vi "run_pharmaBotExpReliability_v0.002.vi"(0 "data in":T9={"daq_ao 1"="Dev1/ao0", "daq_ai 1"="Dev1/ai0", "experiment day folder"=path "C:/multiBot/patcherBot/data/temp", "Multiclamp init error"=0, "Multiclamp Handle Out"=6621140, "sampling rate (Hz)"=20000, "trial name"="t1"}, 5 "auto run?":bool, 7 "which manipulator":T10(ring), 9 "HEK/slice options":enum16{"slice", "HEK"}(ring), 11 "error in":errorcluster, 12 "common cluster":T6, 13 "individual controls in":T5, 14 "images":T3) -> (15 "error out":errorcluster)   [LabVIEW 2015]
uses:
  controls/Load and Save Controls_LV2009.llb/RWC_Actions.ctl
  wc_protocol_v1.003 Folder/whole_cell_protocol/Controls/clamp_profile.ctl
  controls/memtest_def.ctl
  Controls/Data.ctl
  wc_protocol_v1.003 Folder/whole_cell_protocol/Controls/cell_stats-v02.ctl
  pipette cleaning/pressure box/cleaning_soft/controls/actuator_type.ctl
  pipette cleaning/pressure box/cleaning_soft/controls/actuator_cluster.ctl
  machine_vision/coordinate model vis/transform_properties_actuators.ctl
  machine_vision/controls/transform_cluster_actuator.ctl
  controls/NH_method.ctl
  pipette cleaning/pressure box/cleaning_soft/controls/pressure_box_type.ctl
  pipette cleaning/pressure box/cleaning_soft/controls/pressure_box_control.ctl
  multipatch/controls/multipatch_common_controls_v4.ctl
  multipatch/controls/multipatch_individual_controls_v5.ctl
  <vilib>/vision/Image Controls.llb/IMAQ Image.ctl
  multipatch/controls/images_controls.ctl
panel:
  in  "PhaseX Cluster":T1
  out "Running":bool=TRUE
  out "Experiment Done":bool
  in  "Current Position":string
  out "Current Manipulator Position [uM]":i32[](array[numeric]) caption="Current Manipulator Position [um]" format="%.1f"
  in  "ExperimentOptionsCluster":T2
  out "HEK/slice options string":string
  out "config file":path=path "C:/multiBot/patcherBot/autoWCconfigs/autoWC_config_neuron-v07.ini"
  in  "load":bool
  in  "texts":enum32{"status", "comments", "release notes"}(tab)
  out "status":string
  in  "trial comments":string
  in  "release notes":string
  out "cell stats":T7 {"STD" format="%010.2f"; "Variance" format="%010.2f"; "Rt (MOhms)" format="%010.2f"; "tau (ms)" format="%08.2g"; "Cm (pF)" format="%08.2f"; "Ra (MOhms)" format="%010.2f"; "Rm (MOhms)" format="%010.2f"; "Ihold (pA)" format="%010.2f"}
  in  "save":bool
  in  "stop":bool
  in  "output":enum32{"VClamp", "IClamp"}(tab)
  out "Recorded currents (pA)":waveform(dbl)[](graph)
  out "Command steps (mV)":waveform(dbl)[](graph)
  out "Command steps (pA)":waveform(dbl)[](graph)
  out "Recorded voltage (mV)":waveform(dbl)[](graph)
  in  "run":bool
  in  "save as...":bool
  in  "update plots":bool
  in  "protocol creation":T8(tab)
  in  "DEBUG?":bool
  in  "auto WC run trigger":bool
  in  "twitter?":bool
  in  "protocol config":path=path "C:/multiBot/patcherBot/autoWCconfigs/autoWC_config_neuron-v07.ini"
  out "fast comp (pF)":dbl
  out "slow comp (pF)":dbl
  in  "Solution B":string="Wash"
  in  "V2 C Solution8":string="1:1 wash:H20"
  in  "V2 C Solution7":string
  in  "V2 C Solution6":string
  in  "V2 C Solution5":string
  in  "V2 C Solution4":string
  in  "V2 C Solution3":string
  in  "V2 C Solution2":string
  in  "V2 C Solution1":string
  in  "V1 A Solution8":string="1:1 wash:H20"
  in  "V1 A Solution7":string
  in  "V1 A Solution6":string
  in  "V1 A Solution5":string
  in  "V1 A Solution4":string
  in  "V1 A Solution3":string
  in  "V1 A Solution2":string="100uM Glu & 30uM Gly"
  in  "V1 A Solution1":string="Wash"
  in  "repMemTest set":enum32{"Iprot", "Vprot", "Imemtest", "Vmemtest"}(tab)
  out "repMemTest iprot cmd":waveform(dbl)[](graph)
  in  "repMemTest Iprot":T12={"Iclamp in"={"aLevel"=0.0, "aDelta"=0.0, "aDuration"=4000, "bLevel"=-200.0, "bDelta"=100.0, "bDuration"=4000, "cLevel"=0.0, "cDelta"=0.0, "cDuration"=4000}, "# iter"=6, "# reps IC"=1}
  out "repMemTest vprot cmd":waveform(dbl)[](graph)
  in  "repMemTest Vprot":T13={"Vclamp in"={"aLevel"=0.0, "aDelta"=0.0, "aDuration"=40000, "bLevel"=-30.0, "bDelta"=10.0, "bDuration"=40000, "cLevel"=0.0, "cDelta"=0.0, "cDuration"=40000}, "# iter"=8, "# reps VC"=1}
  out "repMemTest imemtest view":waveform(dbl)(graph)
  in  "repMemTest Iclamp memtest":T14={"Samples to Read"=2000, "Rate (Hz)"=20000.0, "Amplitude (mV/pA)"=-50.0, "Offset (mV/pA)"=0.0, "Frequency (Hz)"=10.0, "duty cycle (%)"=50.0, "phase"=0.0} {"phase" format="%.2p"; "duty cycle (%)" format="%0.2f"}
  out "repMemTest vmemtest view":waveform(dbl)(graph)
  in  "repMemTest Vclamp memtest":T14={"Samples to Read"=2000, "Rate (Hz)"=20000.0, "Amplitude (mV/pA)"=10.0, "Offset (mV/pA)"=0.0, "Frequency (Hz)"=10.0, "duty cycle (%)"=50.0, "phase"=-90.0} {"phase" format="%.2p"; "duty cycle (%)" format="%0.2f"}
  in  "wait after init (s)":dbl=0.1
  in  "repMemTest sets":T15={" Iprot"=FALSE, " Vprot"=FALSE, " Imemtest"=FALSE, " Vmemtest"=TRUE}
  in  "wait after repMemTest set (s)":dbl=0.1
  in  "Experimental Phases":T16(tab)
  in  "PhaseA Experiment Option":string(combo)="Single Jump"
  in  "Experiment Selection A":T17(tab)
  in  "Single Jump A":T18={"Which Position to use for Experiment"=enum."Jumper Position B-A", "Start Position (N)"="Jumper Posistion B", "Jump Position (m)"="Jumper Posistion A", "Duration (s)"=10.0, "Delay (s)"=1.0, "Pulse Width (s)"=1.0, "Valve 1 Position"=2, "Valve 2 Position"=2, "Replicates"=1.0, "Vholding (mV)"=-60.0} {"Replicates" min=1.0; "Valve 2 Position" min=1 max=8; "Valve 1 Position" min=1 max=8}
  in  "Solution Change A":T19={"Which Position to use for Experiment"=enum."Jumper Safe Position", "Duration (s)"=0.0, "Delay (s)"=0.0, "Pulse Width (s)"=0.0, "Valve Start Position"=1, "Valve Jump Position"=1, "Replicates"=1.0, "Vholding (mV)"=0.0} {"Replicates" min=1.0; "Valve Jump Position" min=1 max=8; "Valve Start Position" min=1 max=8}
  in  "Voltage Step A":T20={"Which Position to use for Experiment"=enum."Jumper Safe Position", "Duration (s)"=0.0, "Delay (s)"=0.0, "Step Width (s)"=0.0, "Voltage Start (mV)"=1, "Voltage Step (mV)"=1, "Replicates"=1.0, "Voltage End (mV)"=1, "Number of Step"=0.0, "Valve Position"=1, "Vholding (mV)"=0.0} {"Valve Position" min=1 max=8; "Voltage End (mV)" min=1 max=8; "Replicates" min=1.0; "Voltage Step (mV)" min=1 max=8; "Voltage Start (mV)" min=1 max=8}
  in  "Voltage Ramp A":T21={"Which Position to use for Experiment"=enum."Jumper Safe Position", "Duration (s)"=0.0, "Delay (s)"=0.0, "Ramp Slope (mV/s)"=0.0, "Voltage Start (mV)"=1, "Replicates"=1.0, "Voltage End (mV)"=1, "Ramp Duration (s)"=0.0, "Valve Position"=1, "Vholding (mV)"=0.0} {"Valve Position" min=1 max=8; "Voltage End (mV)" min=1 max=8; "Replicates" min=1.0; "Voltage Start (mV)" min=1 max=8}
  in  "Jump Train A":T22={"Which Position to use for Experiment"=enum."Jumper Safe Position", "Start Position (N)"="", "Jump Position (m)"="", "Duration (s)"=0.0, "Delay (s)"=0.0, "Pulse Width (s)"=0.0, "Valve 1 Position"=1, "Valve 2 Position"=1, "Replicates"=1.0, "Pulse Period (s)"=0.0, "Vholding (mV)"=1.0} {"Vholding (mV)" min=1.0; "Replicates" min=1.0; "Valve 2 Position" min=1 max=8; "Valve 1 Position" min=1 max=8}
  in  "Paired Pulse A":T23={"Which Position to use for Experiment"=enum."Jumper Safe Position", "Start Position (N)"="", "Jump Position (m)"="", "Duration (s)"=0.0, "Delay (s)"=0.0, "Pulse Width (s)"=0.0, "Valve 1 Position"=1, "Valve 2 Position"=1, "Replicates"=1.0, "Pulse Delay (s)"=0.0, "Pulse Delta Delay (s)"=0.0, "Vholding (mV)"=0.0} {"Replicates" min=1.0; "Valve 2 Position" min=1 max=8; "Valve 1 Position" min=1 max=8}
  in  "Single Manip Jump A":T24={"Start Position (N)"=enum."Jumper Safe Position", "Duration (s)"=0.0, "Delay (s)"=0.0, "Pulse Width (s)"=0.0, "Valve 1 Position"=1, "Valve 2 Position"=1, "Replicates"=1.0, "Jump Position (m)"=enum."Jumper Safe Position", "Vholding (mV)"=0.0} {"Replicates" min=1.0; "Valve 2 Position" min=1 max=8; "Valve 1 Position" min=1 max=8}
  in  "PhaseB Experiment Option":string(combo)="Single Jump"
  in  "Experiment Selection B":T17(tab)
  in  "Single Jump B":T18={"Which Position to use for Experiment"=enum."Jumper Position B-A", "Start Position (N)"="Jumper Posistion B", "Jump Position (m)"="Jumper Posistion A", "Duration (s)"=10.0, "Delay (s)"=1.0, "Pulse Width (s)"=1.0, "Valve 1 Position"=2, "Valve 2 Position"=2, "Replicates"=1.0, "Vholding (mV)"=40.0} {"Replicates" min=1.0; "Valve 2 Position" min=1 max=8; "Valve 1 Position" min=1 max=8}
  in  "Solution Change B":T19={"Which Position to use for Experiment"=enum."Jumper Safe Position", "Duration (s)"=0.0, "Delay (s)"=0.0, "Pulse Width (s)"=0.0, "Valve Start Position"=1, "Valve Jump Position"=1, "Replicates"=1.0, "Vholding (mV)"=0.0} {"Replicates" min=1.0; "Valve Jump Position" min=1 max=8; "Valve Start Position" min=1 max=8}
  in  "Voltage Step B":T20={"Which Position to use for Experiment"=enum."Jumper Safe Position", "Duration (s)"=0.0, "Delay (s)"=0.0, "Step Width (s)"=0.0, "Voltage Start (mV)"=1, "Voltage Step (mV)"=1, "Replicates"=1.0, "Voltage End (mV)"=1, "Number of Step"=0.0, "Valve Position"=1, "Vholding (mV)"=0.0} {"Valve Position" min=1 max=8; "Voltage End (mV)" min=1 max=8; "Replicates" min=1.0; "Voltage Step (mV)" min=1 max=8; "Voltage Start (mV)" min=1 max=8}
  in  "Voltage Ramp B":T21={"Which Position to use for Experiment"=enum."Jumper Safe Position", "Duration (s)"=0.0, "Delay (s)"=0.0, "Ramp Slope (mV/s)"=0.0, "Voltage Start (mV)"=1, "Replicates"=1.0, "Voltage End (mV)"=1, "Ramp Duration (s)"=0.0, "Valve Position"=1, "Vholding (mV)"=0.0} {"Valve Position" min=1 max=8; "Voltage End (mV)" min=1 max=8; "Replicates" min=1.0; "Voltage Start (mV)" min=1 max=8}
  in  "Jump Train B":T22={"Which Position to use for Experiment"=enum."Jumper Safe Position", "Start Position (N)"="", "Jump Position (m)"="", "Duration (s)"=0.0, "Delay (s)"=0.0, "Pulse Width (s)"=0.0, "Valve 1 Position"=1, "Valve 2 Position"=1, "Replicates"=1.0, "Pulse Period (s)"=0.0, "Vholding (mV)"=1.0} {"Vholding (mV)" min=1.0; "Replicates" min=1.0; "Valve 2 Position" min=1 max=8; "Valve 1 Position" min=1 max=8}
  in  "Paired Pulse B":T23={"Which Position to use for Experiment"=enum."Jumper Safe Position", "Start Position (N)"="", "Jump Position (m)"="", "Duration (s)"=0.0, "Delay (s)"=0.0, "Pulse Width (s)"=0.0, "Valve 1 Position"=1, "Valve 2 Position"=1, "Replicates"=1.0, "Pulse Delay (s)"=0.0, "Pulse Delta Delay (s)"=0.0, "Vholding (mV)"=0.0} {"Replicates" min=1.0; "Valve 2 Position" min=1 max=8; "Valve 1 Position" min=1 max=8}
  in  "Single Manip Jump B":T24={"Start Position (N)"=enum."Jumper Safe Position", "Duration (s)"=0.0, "Delay (s)"=0.0, "Pulse Width (s)"=0.0, "Valve 1 Position"=1, "Valve 2 Position"=1, "Replicates"=1.0, "Jump Position (m)"=enum."Jumper Safe Position", "Vholding (mV)"=0.0} {"Replicates" min=1.0; "Valve 2 Position" min=1 max=8; "Valve 1 Position" min=1 max=8}
  in  "PhaseC Experiment Option":string(combo)="Single Manip Jump"
  in  "Experiment Selection C":T17(tab)=enum."Single Manip Jump"
  in  "Single Jump C":T18={"Which Position to use for Experiment"=enum."Jumper Safe Position", "Start Position (N)"="", "Jump Position (m)"="", "Duration (s)"=0.0, "Delay (s)"=0.0, "Pulse Width (s)"=0.0, "Valve 1 Position"=1, "Valve 2 Position"=1, "Replicates"=1.0, "Vholding (mV)"=0.0} {"Replicates" min=1.0; "Valve 2 Position" min=1 max=8; "Valve 1 Position" min=1 max=8}
  in  "Solution Change C":T19={"Which Position to use for Experiment"=enum."Jumper Safe Position", "Duration (s)"=0.0, "Delay (s)"=0.0, "Pulse Width (s)"=0.0, "Valve Start Position"=1, "Valve Jump Position"=1, "Replicates"=1.0, "Vholding (mV)"=0.0} {"Replicates" min=1.0; "Valve Jump Position" min=1 max=8; "Valve Start Position" min=1 max=8}
  in  "Voltage Step C":T20={"Which Position to use for Experiment"=enum."Jumper Safe Position", "Duration (s)"=0.0, "Delay (s)"=0.0, "Step Width (s)"=0.0, "Voltage Start (mV)"=1, "Voltage Step (mV)"=1, "Replicates"=1.0, "Voltage End (mV)"=1, "Number of Step"=0.0, "Valve Position"=1, "Vholding (mV)"=0.0} {"Valve Position" min=1 max=8; "Voltage End (mV)" min=1 max=8; "Replicates" min=1.0; "Voltage Step (mV)" min=1 max=8; "Voltage Start (mV)" min=1 max=8}
  in  "Voltage Ramp C":T21={"Which Position to use for Experiment"=enum."Jumper Safe Position", "Duration (s)"=0.0, "Delay (s)"=0.0, "Ramp Slope (mV/s)"=0.0, "Voltage Start (mV)"=1, "Replicates"=1.0, "Voltage End (mV)"=1, "Ramp Duration (s)"=0.0, "Valve Position"=1, "Vholding (mV)"=0.0} {"Valve Position" min=1 max=8; "Voltage End (mV)" min=1 max=8; "Replicates" min=1.0; "Voltage Start (mV)" min=1 max=8}
  in  "Jump Train C":T22={"Which Position to use for Experiment"=enum."Jumper Safe Position", "Start Position (N)"="", "Jump Position (m)"="", "Duration (s)"=0.0, "Delay (s)"=0.0, "Pulse Width (s)"=0.0, "Valve 1 Position"=1, "Valve 2 Position"=1, "Replicates"=1.0, "Pulse Period (s)"=0.0, "Vholding (mV)"=1.0} {"Vholding (mV)" min=1.0; "Replicates" min=1.0; "Valve 2 Position" min=1 max=8; "Valve 1 Position" min=1 max=8}
  in  "Paired Pulse C":T23={"Which Position to use for Experiment"=enum."Jumper Safe Position", "Start Position (N)"="", "Jump Position (m)"="", "Duration (s)"=0.0, "Delay (s)"=0.0, "Pulse Width (s)"=0.0, "Valve 1 Position"=1, "Valve 2 Position"=1, "Replicates"=1.0, "Pulse Delay (s)"=0.0, "Pulse Delta Delay (s)"=0.0, "Vholding (mV)"=0.0} {"Replicates" min=1.0; "Valve 2 Position" min=1 max=8; "Valve 1 Position" min=1 max=8}
  in  "Single Manip Jump C":T24={"Start Position (N)"=enum."Jumper Position B", "Duration (s)"=10.0, "Delay (s)"=1.0, "Pulse Width (s)"=1.0, "Valve 1 Position"=2, "Valve 2 Position"=2, "Replicates"=1.0, "Jump Position (m)"=enum."Jumper Position A", "Vholding (mV)"=40.0} {"Replicates" min=1.0; "Valve 2 Position" min=1 max=8; "Valve 1 Position" min=1 max=8}
  in  "PhaseD Experiment Option":string(combo)="Single Manip Jump"
  in  "Experiment Selection D":T17(tab)=enum."Single Manip Jump"
  in  "Single Jump D":T18={"Which Position to use for Experiment"=enum."Jumper Safe Position", "Start Position (N)"="", "Jump Position (m)"="", "Duration (s)"=0.0, "Delay (s)"=0.0, "Pulse Width (s)"=0.0, "Valve 1 Position"=1, "Valve 2 Position"=1, "Replicates"=1.0, "Vholding (mV)"=0.0} {"Replicates" min=1.0; "Valve 2 Position" min=1 max=8; "Valve 1 Position" min=1 max=8}
  in  "Solution Change D":T19={"Which Position to use for Experiment"=enum."Jumper Safe Position", "Duration (s)"=0.0, "Delay (s)"=0.0, "Pulse Width (s)"=0.0, "Valve Start Position"=1, "Valve Jump Position"=1, "Replicates"=1.0, "Vholding (mV)"=0.0} {"Replicates" min=1.0; "Valve Jump Position" min=1 max=8; "Valve Start Position" min=1 max=8}
  in  "Voltage Step D":T20={"Which Position to use for Experiment"=enum."Jumper Safe Position", "Duration (s)"=0.0, "Delay (s)"=0.0, "Step Width (s)"=0.0, "Voltage Start (mV)"=1, "Voltage Step (mV)"=1, "Replicates"=1.0, "Voltage End (mV)"=1, "Number of Step"=0.0, "Valve Position"=1, "Vholding (mV)"=0.0} {"Valve Position" min=1 max=8; "Voltage End (mV)" min=1 max=8; "Replicates" min=1.0; "Voltage Step (mV)" min=1 max=8; "Voltage Start (mV)" min=1 max=8}
  in  "Voltage Ramp D":T21={"Which Position to use for Experiment"=enum."Jumper Safe Position", "Duration (s)"=0.0, "Delay (s)"=0.0, "Ramp Slope (mV/s)"=0.0, "Voltage Start (mV)"=1, "Replicates"=1.0, "Voltage End (mV)"=1, "Ramp Duration (s)"=0.0, "Valve Position"=1, "Vholding (mV)"=0.0} {"Valve Position" min=1 max=8; "Voltage End (mV)" min=1 max=8; "Replicates" min=1.0; "Voltage Start (mV)" min=1 max=8}
  in  "Jump Train D":T22={"Which Position to use for Experiment"=enum."Jumper Safe Position", "Start Position (N)"="", "Jump Position (m)"="", "Duration (s)"=0.0, "Delay (s)"=0.0, "Pulse Width (s)"=0.0, "Valve 1 Position"=1, "Valve 2 Position"=1, "Replicates"=1.0, "Pulse Period (s)"=0.0, "Vholding (mV)"=1.0} {"Vholding (mV)" min=1.0; "Replicates" min=1.0; "Valve 2 Position" min=1 max=8; "Valve 1 Position" min=1 max=8}
  in  "Paired Pulse D":T23={"Which Position to use for Experiment"=enum."Jumper Safe Position", "Start Position (N)"="", "Jump Position (m)"="", "Duration (s)"=0.0, "Delay (s)"=0.0, "Pulse Width (s)"=0.0, "Valve 1 Position"=1, "Valve 2 Position"=1, "Replicates"=1.0, "Pulse Delay (s)"=0.0, "Pulse Delta Delay (s)"=0.0, "Vholding (mV)"=0.0} {"Replicates" min=1.0; "Valve 2 Position" min=1 max=8; "Valve 1 Position" min=1 max=8}
  in  "Single Manip Jump D":T24={"Start Position (N)"=enum."Jumper Position B", "Duration (s)"=10.0, "Delay (s)"=1.0, "Pulse Width (s)"=1.0, "Valve 1 Position"=2, "Valve 2 Position"=2, "Replicates"=1.0, "Jump Position (m)"=enum."Jumper Position A", "Vholding (mV)"=-60.0} {"Replicates" min=1.0; "Valve 2 Position" min=1 max=8; "Valve 1 Position" min=1 max=8}
  in  "PhaseE Experiment Option":string(combo)="Single Manip Jump"
  in  "Experiment Selection E":T17(tab)=enum."Single Manip Jump"
  in  "Single Jump E":T18={"Which Position to use for Experiment"=enum."Jumper Safe Position", "Start Position (N)"="", "Jump Position (m)"="", "Duration (s)"=0.0, "Delay (s)"=0.0, "Pulse Width (s)"=0.0, "Valve 1 Position"=1, "Valve 2 Position"=1, "Replicates"=1.0, "Vholding (mV)"=0.0} {"Replicates" min=1.0; "Valve 2 Position" min=1 max=8; "Valve 1 Position" min=1 max=8}
  in  "Solution Change E":T19={"Which Position to use for Experiment"=enum."Jumper Safe Position", "Duration (s)"=0.0, "Delay (s)"=0.0, "Pulse Width (s)"=0.0, "Valve Start Position"=1, "Valve Jump Position"=1, "Replicates"=1.0, "Vholding (mV)"=0.0} {"Replicates" min=1.0; "Valve Jump Position" min=1 max=8; "Valve Start Position" min=1 max=8}
  in  "Voltage Step E":T20={"Which Position to use for Experiment"=enum."Jumper Safe Position", "Duration (s)"=0.0, "Delay (s)"=0.0, "Step Width (s)"=0.0, "Voltage Start (mV)"=1, "Voltage Step (mV)"=1, "Replicates"=1.0, "Voltage End (mV)"=1, "Number of Step"=0.0, "Valve Position"=1, "Vholding (mV)"=0.0} {"Valve Position" min=1 max=8; "Voltage End (mV)" min=1 max=8; "Replicates" min=1.0; "Voltage Step (mV)" min=1 max=8; "Voltage Start (mV)" min=1 max=8}
  in  "Voltage Ramp E":T21={"Which Position to use for Experiment"=enum."Jumper Safe Position", "Duration (s)"=0.0, "Delay (s)"=0.0, "Ramp Slope (mV/s)"=0.0, "Voltage Start (mV)"=1, "Replicates"=1.0, "Voltage End (mV)"=1, "Ramp Duration (s)"=0.0, "Valve Position"=1, "Vholding (mV)"=0.0} {"Valve Position" min=1 max=8; "Voltage End (mV)" min=1 max=8; "Replicates" min=1.0; "Voltage Start (mV)" min=1 max=8}
  in  "Jump Train E":T22={"Which Position to use for Experiment"=enum."Jumper Safe Position", "Start Position (N)"="", "Jump Position (m)"="", "Duration (s)"=0.0, "Delay (s)"=0.0, "Pulse Width (s)"=0.0, "Valve 1 Position"=1, "Valve 2 Position"=1, "Replicates"=1.0, "Pulse Period (s)"=0.0, "Vholding (mV)"=1.0} {"Vholding (mV)" min=1.0; "Replicates" min=1.0; "Valve 2 Position" min=1 max=8; "Valve 1 Position" min=1 max=8}
  in  "Paired Pulse E":T23={"Which Position to use for Experiment"=enum."Jumper Safe Position", "Start Position (N)"="", "Jump Position (m)"="", "Duration (s)"=0.0, "Delay (s)"=0.0, "Pulse Width (s)"=0.0, "Valve 1 Position"=1, "Valve 2 Position"=1, "Replicates"=1.0, "Pulse Delay (s)"=0.0, "Pulse Delta Delay (s)"=0.0, "Vholding (mV)"=0.0} {"Replicates" min=1.0; "Valve 2 Position" min=1 max=8; "Valve 1 Position" min=1 max=8}
  in  "Single Manip Jump E":T24={"Start Position (N)"=enum."Jumper Position B", "Duration (s)"=10.0, "Delay (s)"=1.0, "Pulse Width (s)"=1.0, "Valve 1 Position"=2, "Valve 2 Position"=2, "Replicates"=1.0, "Jump Position (m)"=enum."Jumper Position o-A", "Vholding (mV)"=-60.0} {"Replicates" min=1.0; "Valve 2 Position" min=1 max=8; "Valve 1 Position" min=1 max=8}
  in  "PhaseF Experiment Option":string(combo)="Single Jump"
  in  "Experiment Selection F":T17(tab)
  in  "Single Jump F":T18={"Which Position to use for Experiment"=enum."Jumper Position B-A", "Start Position (N)"="Jumper Posistion B", "Jump Position (m)"="Jumper Posistion A", "Duration (s)"=10.0, "Delay (s)"=1.0, "Pulse Width (s)"=1.0, "Valve 1 Position"=2, "Valve 2 Position"=2, "Replicates"=1.0, "Vholding (mV)"=-60.0} {"Replicates" min=1.0; "Valve 2 Position" min=1 max=8; "Valve 1 Position" min=1 max=8}
  in  "Solution Change F":T19={"Which Position to use for Experiment"=enum."Jumper Safe Position", "Duration (s)"=0.0, "Delay (s)"=0.0, "Pulse Width (s)"=0.0, "Valve Start Position"=1, "Valve Jump Position"=1, "Replicates"=1.0, "Vholding (mV)"=0.0} {"Replicates" min=1.0; "Valve Jump Position" min=1 max=8; "Valve Start Position" min=1 max=8}
  in  "Voltage Step F":T20={"Which Position to use for Experiment"=enum."Jumper Safe Position", "Duration (s)"=0.0, "Delay (s)"=0.0, "Step Width (s)"=0.0, "Voltage Start (mV)"=1, "Voltage Step (mV)"=1, "Replicates"=1.0, "Voltage End (mV)"=1, "Number of Step"=0.0, "Valve Position"=1, "Vholding (mV)"=0.0} {"Valve Position" min=1 max=8; "Voltage End (mV)" min=1 max=8; "Replicates" min=1.0; "Voltage Step (mV)" min=1 max=8; "Voltage Start (mV)" min=1 max=8}
  in  "Voltage Ramp F":T21={"Which Position to use for Experiment"=enum."Jumper Safe Position", "Duration (s)"=0.0, "Delay (s)"=0.0, "Ramp Slope (mV/s)"=0.0, "Voltage Start (mV)"=1, "Replicates"=1.0, "Voltage End (mV)"=1, "Ramp Duration (s)"=0.0, "Valve Position"=1, "Vholding (mV)"=0.0} {"Valve Position" min=1 max=8; "Voltage End (mV)" min=1 max=8; "Replicates" min=1.0; "Voltage Start (mV)" min=1 max=8}
  in  "Jump Train F":T22={"Which Position to use for Experiment"=enum."Jumper Safe Position", "Start Position (N)"="", "Jump Position (m)"="", "Duration (s)"=0.0, "Delay (s)"=0.0, "Pulse Width (s)"=0.0, "Valve 1 Position"=1, "Valve 2 Position"=1, "Replicates"=1.0, "Pulse Period (s)"=0.0, "Vholding (mV)"=1.0} {"Vholding (mV)" min=1.0; "Replicates" min=1.0; "Valve 2 Position" min=1 max=8; "Valve 1 Position" min=1 max=8}
  in  "Paired Pulse F":T23={"Which Position to use for Experiment"=enum."Jumper Safe Position", "Start Position (N)"="", "Jump Position (m)"="", "Duration (s)"=0.0, "Delay (s)"=0.0, "Pulse Width (s)"=0.0, "Valve 1 Position"=1, "Valve 2 Position"=1, "Replicates"=1.0, "Pulse Delay (s)"=0.0, "Pulse Delta Delay (s)"=0.0, "Vholding (mV)"=0.0} {"Replicates" min=1.0; "Valve 2 Position" min=1 max=8; "Valve 1 Position" min=1 max=8}
  in  "Single Manip Jump F":T24={"Start Position (N)"=enum."Jumper Safe Position", "Duration (s)"=0.0, "Delay (s)"=0.0, "Pulse Width (s)"=0.0, "Valve 1 Position"=1, "Valve 2 Position"=1, "Replicates"=1.0, "Jump Position (m)"=enum."Jumper Safe Position", "Vholding (mV)"=0.0} {"Replicates" min=1.0; "Valve 2 Position" min=1 max=8; "Valve 1 Position" min=1 max=8}
  in  "ending set":enum32{"Iprot", "Vprot", "Imemtest", "Vmemtest"}(tab)
  in  "holding memtest":bool=TRUE
  in  "holding set":enum32{"VClamp", "IClamp"}(tab)
  out "holding vmemtest cmd":waveform(dbl)(graph)
  in  "holding Vclamp memtest":T14={"Samples to Read"=2000, "Rate (Hz)"=20000.0, "Amplitude (mV/pA)"=10.0, "Offset (mV/pA)"=0.0, "Frequency (Hz)"=10.0, "duty cycle (%)"=50.0, "phase"=-90.0} {"phase" format="%.2p"; "duty cycle (%)" format="%0.2f"}
  out "holding imemtest cmd":waveform(dbl)(graph)
  in  "holding Iclamp memtest":T14={"Samples to Read"=2000, "Rate (Hz)"=20000.0, "Amplitude (mV/pA)"=-50.0, "Offset (mV/pA)"=0.0, "Frequency (Hz)"=10.0, "duty cycle (%)"=50.0, "phase"=0.0} {"phase" format="%.2p"; "duty cycle (%)" format="%0.2f"}
  # "IClamp step protocol"
  # "x"
  # "VClamp step protocol"
  # "x"
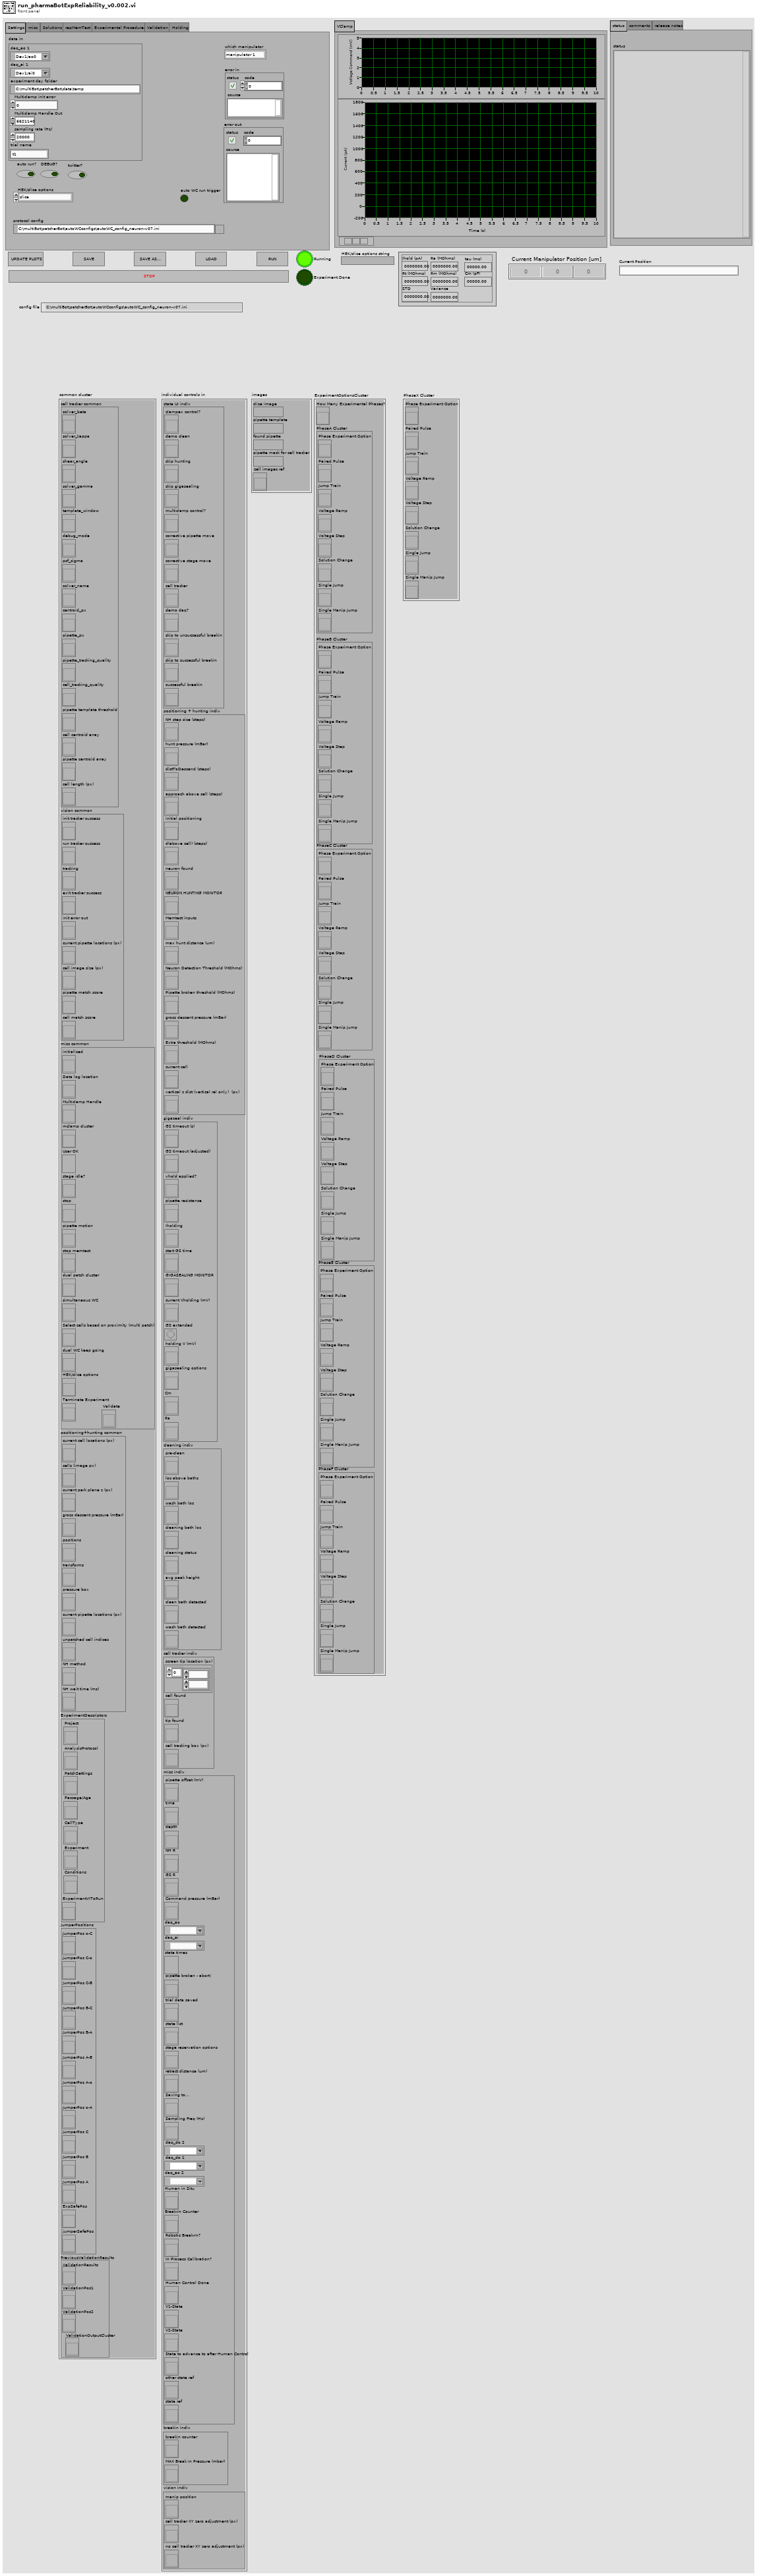
[diagram p1: front panel]
types:
  T1 = cluster{"Phase Experiment Option":refnum<vi>, "Paired Pulse":refnum<vi>, "Jump Train":refnum<vi>, "Voltage Ramp":refnum<vi>, "Voltage Step":refnum<vi>, "Solution Change":refnum<vi>, "Single Jump":refnum<vi>, "Single Manip Jump":refnum<vi>}
  T2 = cluster{"How Many Experimental Phases?":refnum<vi>, "PhaseA Cluster":cluster{"Phase Experiment Option":refnum<vi>, "Paired Pulse":refnum<vi>, "Jump Train":refnum<vi>, "Voltage Ramp":refnum<vi>, "Voltage Step":refnum<vi>, "Solution Change":refnum<vi>, "Single Jump":refnum<vi>, "Single Manip Jump":refnum<vi>}, "PhaseB Cluster":cluster{"Phase Experiment Option":refnum<vi>, "Paired Pulse":refnum<vi>, "Jump Train":refnum<vi>, "Voltage Ramp":refnum<vi>, "Voltage Step":refnum<vi>, "Solution Change":refnum<vi>, "Single Jump":refnum<vi>, "Single Manip Jump":refnum<vi>}, "PhaseC Cluster":cluster{"Phase Experiment Option":refnum<vi>, "Paired Pulse":refnum<vi>, "Jump Train":refnum<vi>, "Voltage Ramp":refnum<vi>, "Voltage Step":refnum<vi>, "Solution Change":refnum<vi>, "Single Jump":refnum<vi>, "Single Manip Jump":refnum<vi>}, "PhaseD Cluster":cluster{"Phase Experiment Option":refnum<vi>, "Paired Pulse":refnum<vi>, "Jump Train":refnum<vi>, "Voltage Ramp":refnum<vi>, "Voltage Step":refnum<vi>, "Solution Change":refnum<vi>, "Single Jump":refnum<vi>, "Single Manip Jump":refnum<vi>}, "PhaseE Cluster":cluster{"Phase Experiment Option":refnum<vi>, "Paired Pulse":refnum<vi>, "Jump Train":refnum<vi>, "Voltage Ramp":refnum<vi>, "Voltage Step":refnum<vi>, "Solution Change":refnum<vi>, "Single Jump":refnum<vi>, "Single Manip Jump":refnum<vi>}, "PhaseF Cluster":cluster{"Phase Experiment Option":refnum<vi>, "Paired Pulse":refnum<vi>, "Jump Train":refnum<vi>, "Voltage Ramp":refnum<vi>, "Voltage Step":refnum<vi>, "Solution Change":refnum<vi>, "Single Jump":refnum<vi>, "Single Manip Jump":refnum<vi>}}
  T3 = typedef "images_controls.ctl" = cluster{"slice image":T4, "pipette template":T4, "found pipette":T4, "pipette mask for cell tracker":T4, "cell images ref":refnum<vi>}
  T4 = typedef "IMAQ Image.ctl" = refnum<image>
  T5 = typedef "multipatch_individual_controls_v5.ctl" = cluster{"state UI indiv":cluster{"clampex control?":refnum<vi>, "demo clean":refnum<vi>, "skip hunting":refnum<vi>, "skip gigasealing":refnum<vi>, "multiclamp control?":refnum<vi>, "corrective pipette move":refnum<vi>, "corrective stage move":refnum<vi>, "cell tracker":refnum<vi>, "demo daq?":refnum<vi>, "skip to unsuccessful breakin":refnum<vi>, "skip to successful breakin":refnum<vi>, "successful breakin":refnum<vi>}, "positioning + hunting indiv":cluster{"NH step size (steps)":refnum<vi>, "hunt pressure (mBar)":refnum<vi>, "distToDescend (steps)":refnum<vi>, "approach above cell (steps)":refnum<vi>, "initial positioning":refnum<vi>, "d(above cell) (steps)":refnum<vi>, "neuron found":refnum<vi>, "NEURON HUNTING MONITOR":refnum<vi>, "Memtest inputs":refnum<vi>, "max hunt distance (um)":refnum<vi>, "Neuron Detection Threshold (MOhms)":refnum<vi>, "Pipette broken threshold (MOhms)":refnum<vi>, "gross descent pressure (mBar)":refnum<vi>, "Extra threshold (MOhms)":refnum<vi>, "current cell":refnum<vi>, "vertical z dist (vertical rel only)  (px)":refnum<vi>}, "gigaseal indiv":cluster{"GS timeout (s)":refnum<vi>, "GS timeout (adjusted)":refnum<vi>, "vhold applied?":refnum<vi>, "pipette resistance":refnum<vi>, "Iholding":refnum<vi>, "start GS time":refnum<vi>, "GIGASEALING MONITOR":refnum<vi>, "current Vholding (mV)":refnum<vi>, "GS extended":refnum<vi>, "holding V (mV)":refnum<vi>, "gigasealing options":refnum<vi>, "Cm":refnum<vi>, "Ra ":refnum<vi>}, "cleaning indiv":cluster{"pre-clean":refnum<vi>, "loc above baths":refnum<vi>, "wash bath loc":refnum<vi>, "cleaning bath loc":refnum<vi>, "cleaning status":refnum<vi>, "avg peak height":refnum<vi>, "clean bath detected":refnum<vi>, "wash bath detected":refnum<vi>}, "cell tracker indiv":cluster{"screen tip location (px)":refnum<vi>, "cell found":refnum<vi>, "tip found":refnum<vi>, "cell tracking box (px)":refnum<vi>}, "misc indiv":cluster{"pipette offset (mV)":refnum<vi>, "time":refnum<vi>, "depth":refnum<vi>, "NH R":refnum<vi>, "GS R":refnum<vi>, "Command pressure (mBar)":refnum<vi>, "daq_ao":tag, "daq_ai":tag, "state times":refnum<vi>, "pipette broken - abort!":refnum<vi>, "trial data saved":refnum<vi>, "state list":refnum<vi>, "stage reservation options":refnum<vi>, "retract distance (um)":refnum<vi>, "Saving to...":refnum<vi>, "Sampling Freq (Hz)":refnum<vi>, "daq_do 2":tag, "daq_do 1":tag, "daq_ao 2":tag, "Human in Situ":refnum<vi>, "Break-In Counter":refnum<vi>, "Robotic Break-In?":refnum<vi>, "In Process Calibration?":refnum<vi>, "Human Control Done":refnum<vi>, "V1-State":refnum<vi>, "V2-State":refnum<vi>, "State to advance to after Human Control":refnum<vi>, "other state ref":refnum<vi>, "state ref":refnum<vi>}, "breakin indiv":cluster{"breakin counter":refnum<vi>, "MAX Break In Pressure (mbar)":refnum<vi>}, "vision indiv":cluster{"manip position":refnum<vi>, "cell tracker XY zero adjustment (px)":refnum<vi>, "no cell tracker XY zero adjustment (px)":refnum<vi>}}
  T6 = typedef "multipatch_common_controls_v4.ctl" = cluster{"cell tracker common":cluster{"solver_beta":refnum<vi>, "solver_kappa":refnum<vi>, "shear_angle":refnum<vi>, "solver_gamma":refnum<vi>, "template_window":refnum<vi>, "debug_mode":refnum<vi>, "psf_sigma":refnum<vi>, "solver_name":refnum<vi>, "centroid_px":refnum<vi>, "pipette_px":refnum<vi>, "pipette_tracking_quality":refnum<vi>, "cell_tracking_quality":refnum<vi>, "pipette template threshold":refnum<vi>, "cell centroid array":refnum<vi>, "pipette centroid array":refnum<vi>, "cell length (px)":refnum<vi>}, "vision common":cluster{"init tracker success":refnum<vi>, "run tracker success":refnum<vi>, "tracking":refnum<vi>, "exit tracker success":refnum<vi>, "init error out":refnum<vi>, "current pipette locations (px)":refnum<vi>, "cell image size (px)":refnum<vi>, "pipette match score":refnum<vi>, "cell match score":refnum<vi>}, "misc common":cluster{"initialized":refnum<vi>, "Data log location":refnum<vi>, "Multiclamp Handle":refnum<vi>, "mclamp cluster":refnum<vi>, "User OK":refnum<vi>, "stage idle?":refnum<vi>, "stop":refnum<vi>, "pipette motion":refnum<vi>, "stop memtest":refnum<vi>, "dual patch cluster":refnum<vi>, "simultaneous WC":refnum<vi>, "Select cells based on proximity (multi patch)":refnum<vi>, "dual WC keep going":refnum<vi>, "HEK/slice options":refnum<vi>, "Terminate Experiment":refnum<vi>, "Validate":refnum<vi>}, "positioning+hunting common":cluster{"current cell locations (px)":refnum<vi>, "cells (image px)":refnum<vi>, "current park plane z (px)":refnum<vi>, "gross descent pressure (mBar)":refnum<vi>, "positions":refnum<vi>, "transforms":refnum<vi>, "pressure box":refnum<vi>, "current pipette locations (px)":refnum<vi>, "unpatched cell indices":refnum<vi>, "NH method":refnum<vi>, "NH wait time (ms)":refnum<vi>}, "ExperimentDescriptors":cluster{"Project":refnum<vi>, "AnalysisProtocol":refnum<vi>, "PatchSettings":refnum<vi>, "Passage/Age":refnum<vi>, "CellType":refnum<vi>, "Experiment":refnum<vi>, "Conditions":refnum<vi>, "ExperimentVIToRun":refnum<vi>}, "JumperPositions":cluster{"JumperPos o-C":refnum<vi>, "JumperPos C-o":refnum<vi>, "JumperPos C-B":refnum<vi>, "JumperPos B-C":refnum<vi>, "JumperPos B-A":refnum<vi>, "JumperPos A-B":refnum<vi>, "JumperPos A-o":refnum<vi>, "JumperPos o-A":refnum<vi>, "JumperPos C":refnum<vi>, "JumperPos B":refnum<vi>, "JumperPos A":refnum<vi>, "ExpSafePos":refnum<vi>, "jumperSafePos":refnum<vi>}, "PreviousValidationResults":cluster{"ValidationResults":refnum<vi>, "ValidationPos1":refnum<vi>, "ValidationPos2":refnum<vi>, "ValidationOutputCluster":refnum<vi>}}
  T7 = typedef "cell_stats-v02.ctl" = cluster{"Ihold (pA)":dbl, "Rm (MOhms)":dbl, "Ra (MOhms)":dbl, "Cm (pF)":dbl, "tau (ms)":dbl, "Rt (MOhms)":dbl, "Variance":dbl, "STD":dbl}
  T8 = enum32{"Settings", "misc", "Solutions", "repMemTest", "Experimental Procedures", "Validation", "Holding"}
  T9 = typedef "Data.ctl" = cluster{"daq_ao 1":tag, "daq_ai 1":tag, "experiment day folder":path, "Multiclamp init error":i32, "Multiclamp Handle Out":u32, "sampling rate (Hz)":i32, "trial name":string}
  T10 = enum16{"manipulator 1", "manipulator 2", "manipulator 3", "manipulator 4"}
  T11 = typedef "clamp_profile.ctl" = cluster{"aLevel":dbl, "aDelta":dbl, "aDuration":i32, "bLevel":dbl, "bDelta":dbl, "bDuration":i32, "cLevel":dbl, "cDelta":dbl, "cDuration":i32}
  T12 = cluster{"Iclamp in":T11, "# iter":i32, "# reps IC":i32}
  T13 = cluster{"Vclamp in":T11, "# iter":i32, "# reps VC":i32}
  T14 = typedef "memtest_def.ctl" = cluster{"Samples to Read":i32, "Rate (Hz)":dbl, "Amplitude (mV/pA)":dbl, "Offset (mV/pA)":dbl, "Frequency (Hz)":dbl, "duty cycle (%)":dbl, "phase":dbl}
  T15 = cluster{" Iprot":bool, " Vprot":bool, " Imemtest":bool, " Vmemtest":bool}
  T16 = enum32{"PhaseA", "PhaseB", "PhaseC", "PhaseD", "PhaseE", "PhaseF", "PhaseG", "PhaseH", "PhaseI", "PhaseJ", "PhaseK", "PhaseL", "PhaseM", "PhaseN"}
  T17 = enum32{"Single Jump", "Solution Change", "Voltage Step", "Voltage Ramp", "Jump Train", "Paired Pulse", "Single Manip Jump"}
  T18 = cluster{"Which Position to use for Experiment":enum16{"Jumper Safe Position", "Experiment Safe Position", "Jumper Position A", "Jumper Position B", "Jumper Position C", "Jumper Position o-A", "Jumper Position A-o", "Jumper Position A-B", "Jumper Position B-A", "Jumper Position B-C", "Jumper Position C-B", "Jumper Position C-o", "Jumper Position o-C"}, "Start Position (N)":string, "Jump Position (m)":string, "Duration (s)":dbl, "Delay (s)":dbl, "Pulse Width (s)":dbl, "Valve 1 Position":i16, "Valve 2 Position":i16, "Replicates":dbl, "Vholding (mV)":dbl}
  T19 = cluster{"Which Position to use for Experiment":enum16{"Jumper Safe Position", "Experiment Safe Position", "Jumper Position A", "Jumper Position B", "Jumper Position C", "Jumper Position o-A", "Jumper Position A-o", "Jumper Position A-B", "Jumper Position B-A", "Jumper Position B-C", "Jumper Position C-B", "Jumper Position C-o", "Jumper Position o-C"}, "Duration (s)":dbl, "Delay (s)":dbl, "Pulse Width (s)":dbl, "Valve Start Position":i16, "Valve Jump Position":i16, "Replicates":dbl, "Vholding (mV)":dbl}
  T20 = cluster{"Which Position to use for Experiment":enum16{"Jumper Safe Position", "Experiment Safe Position", "Jumper Position A", "Jumper Position B", "Jumper Position C", "Jumper Position o-A", "Jumper Position A-o", "Jumper Position A-B", "Jumper Position B-A", "Jumper Position B-C", "Jumper Position C-B", "Jumper Position C-o", "Jumper Position o-C"}, "Duration (s)":dbl, "Delay (s)":dbl, "Step Width (s)":dbl, "Voltage Start (mV)":i16, "Voltage Step (mV)":i16, "Replicates":dbl, "Voltage End (mV)":i16, "Number of Step":dbl, "Valve Position":i16, "Vholding (mV)":dbl}
  T21 = cluster{"Which Position to use for Experiment":enum16{"Jumper Safe Position", "Experiment Safe Position", "Jumper Position A", "Jumper Position B", "Jumper Position C", "Jumper Position o-A", "Jumper Position A-o", "Jumper Position A-B", "Jumper Position B-A", "Jumper Position B-C", "Jumper Position C-B", "Jumper Position C-o", "Jumper Position o-C"}, "Duration (s)":dbl, "Delay (s)":dbl, "Ramp Slope (mV/s)":dbl, "Voltage Start (mV)":i16, "Replicates":dbl, "Voltage End (mV)":i16, "Ramp Duration (s)":dbl, "Valve Position":i16, "Vholding (mV)":dbl}
  T22 = cluster{"Which Position to use for Experiment":enum16{"Jumper Safe Position", "Experiment Safe Position", "Jumper Position A", "Jumper Position B", "Jumper Position C", "Jumper Position o-A", "Jumper Position A-o", "Jumper Position A-B", "Jumper Position B-A", "Jumper Position B-C", "Jumper Position C-B", "Jumper Position C-o", "Jumper Position o-C"}, "Start Position (N)":string, "Jump Position (m)":string, "Duration (s)":dbl, "Delay (s)":dbl, "Pulse Width (s)":dbl, "Valve 1 Position":i16, "Valve 2 Position":i16, "Replicates":dbl, "Pulse Period (s)":dbl, "Vholding (mV)":dbl}
  T23 = cluster{"Which Position to use for Experiment":enum16{"Jumper Safe Position", "Experiment Safe Position", "Jumper Position A", "Jumper Position B", "Jumper Position C", "Jumper Position o-A", "Jumper Position A-o", "Jumper Position A-B", "Jumper Position B-A", "Jumper Position B-C", "Jumper Position C-B", "Jumper Position C-o", "Jumper Position o-C"}, "Start Position (N)":string, "Jump Position (m)":string, "Duration (s)":dbl, "Delay (s)":dbl, "Pulse Width (s)":dbl, "Valve 1 Position":i16, "Valve 2 Position":i16, "Replicates":dbl, "Pulse Delay (s)":dbl, "Pulse Delta Delay (s)":dbl, "Vholding (mV)":dbl}
  T24 = cluster{"Start Position (N)":enum16{"Jumper Safe Position", "Experiment Safe Position", "Jumper Position A", "Jumper Position B", "Jumper Position C", "Jumper Position o-A", "Jumper Position A-o", "Jumper Position A-B", "Jumper Position B-A", "Jumper Position B-C", "Jumper Position C-B", "Jumper Position C-o", "Jumper Position o-C"}, "Duration (s)":dbl, "Delay (s)":dbl, "Pulse Width (s)":dbl, "Valve 1 Position":i16, "Valve 2 Position":i16, "Replicates":dbl, "Jump Position (m)":enum16{"Jumper Safe Position", "Experiment Safe Position", "Jumper Position A", "Jumper Position B", "Jumper Position C", "Jumper Position o-A", "Jumper Position A-o", "Jumper Position A-B", "Jumper Position B-A", "Jumper Position B-C", "Jumper Position C-B", "Jumper Position C-o", "Jumper Position o-C"}, "Vholding (mV)":dbl}
  T25 = typedef "RWC_Actions.ctl" = enum16{"Read", "Write", "Read and Create"}
  T26 = typedef "pressure_box_control.ctl" = cluster{"Pressure box COM":refnum<visa-resource-name>, "pressure box type":T27, "High pos pressure (mBar)":dbl, "Low pos pressure (mBar)":dbl, "Vacuum pressure (mBar)":dbl, "calibration":enum16{"PA_vacPump", "PA_venturi", "Neuromatics", "ilyaRig", "mightenRig"}}
  T27 = typedef "pressure_box_type.ctl" = enum16{"Neuromatics", "ProportionAir", "Demo box", "N-ProportionAir"}
  T28 = enum16{"Jumper Safe Position", "Experiment Safe Position", "Jumper Position A", "Jumper Position B", "Jumper Position C", "Jumper Position o-A", "Jumper Position A-o", "Jumper Position A-B", "Jumper Position B-A", "Jumper Position B-C", "Jumper Position C-B", "Jumper Position C-o", "Jumper Position o-C"}
  T29 = typedef "transform_cluster_actuator.ctl" = cluster{"s":refnum<vi>, "manip 1":refnum<vi>, "manip 2":refnum<vi>, "manip 3":refnum<vi>, "manip 4":refnum<vi>}
  T30 = typedef "transform_properties_actuators.ctl" = cluster{"theta (deg)":dbl, "X sc factor (px/step)":dbl, "Y sc factor (px/step)":dbl, "zero loc (x,y,z)":dbl[], "flip y?":bool, "flip x?":bool, "gamma (deg)":dbl, "flip z?":bool, "Z sc factor (px/step)":dbl, "actuator":T31, "safe space (steps)":i32[]}
  T31 = typedef "actuator_cluster.ctl" = cluster{"Actuator COM":refnum<visa-resource-name>, "Actuator type":T32}
  T32 = typedef "actuator_type.ctl" = enum16{"Scientifica", "Sutter", "Demo", "Off"}
  T33 = enum16{"open", "replace", "create", "open or create", "replace or create", "replace or create with confirmation"}
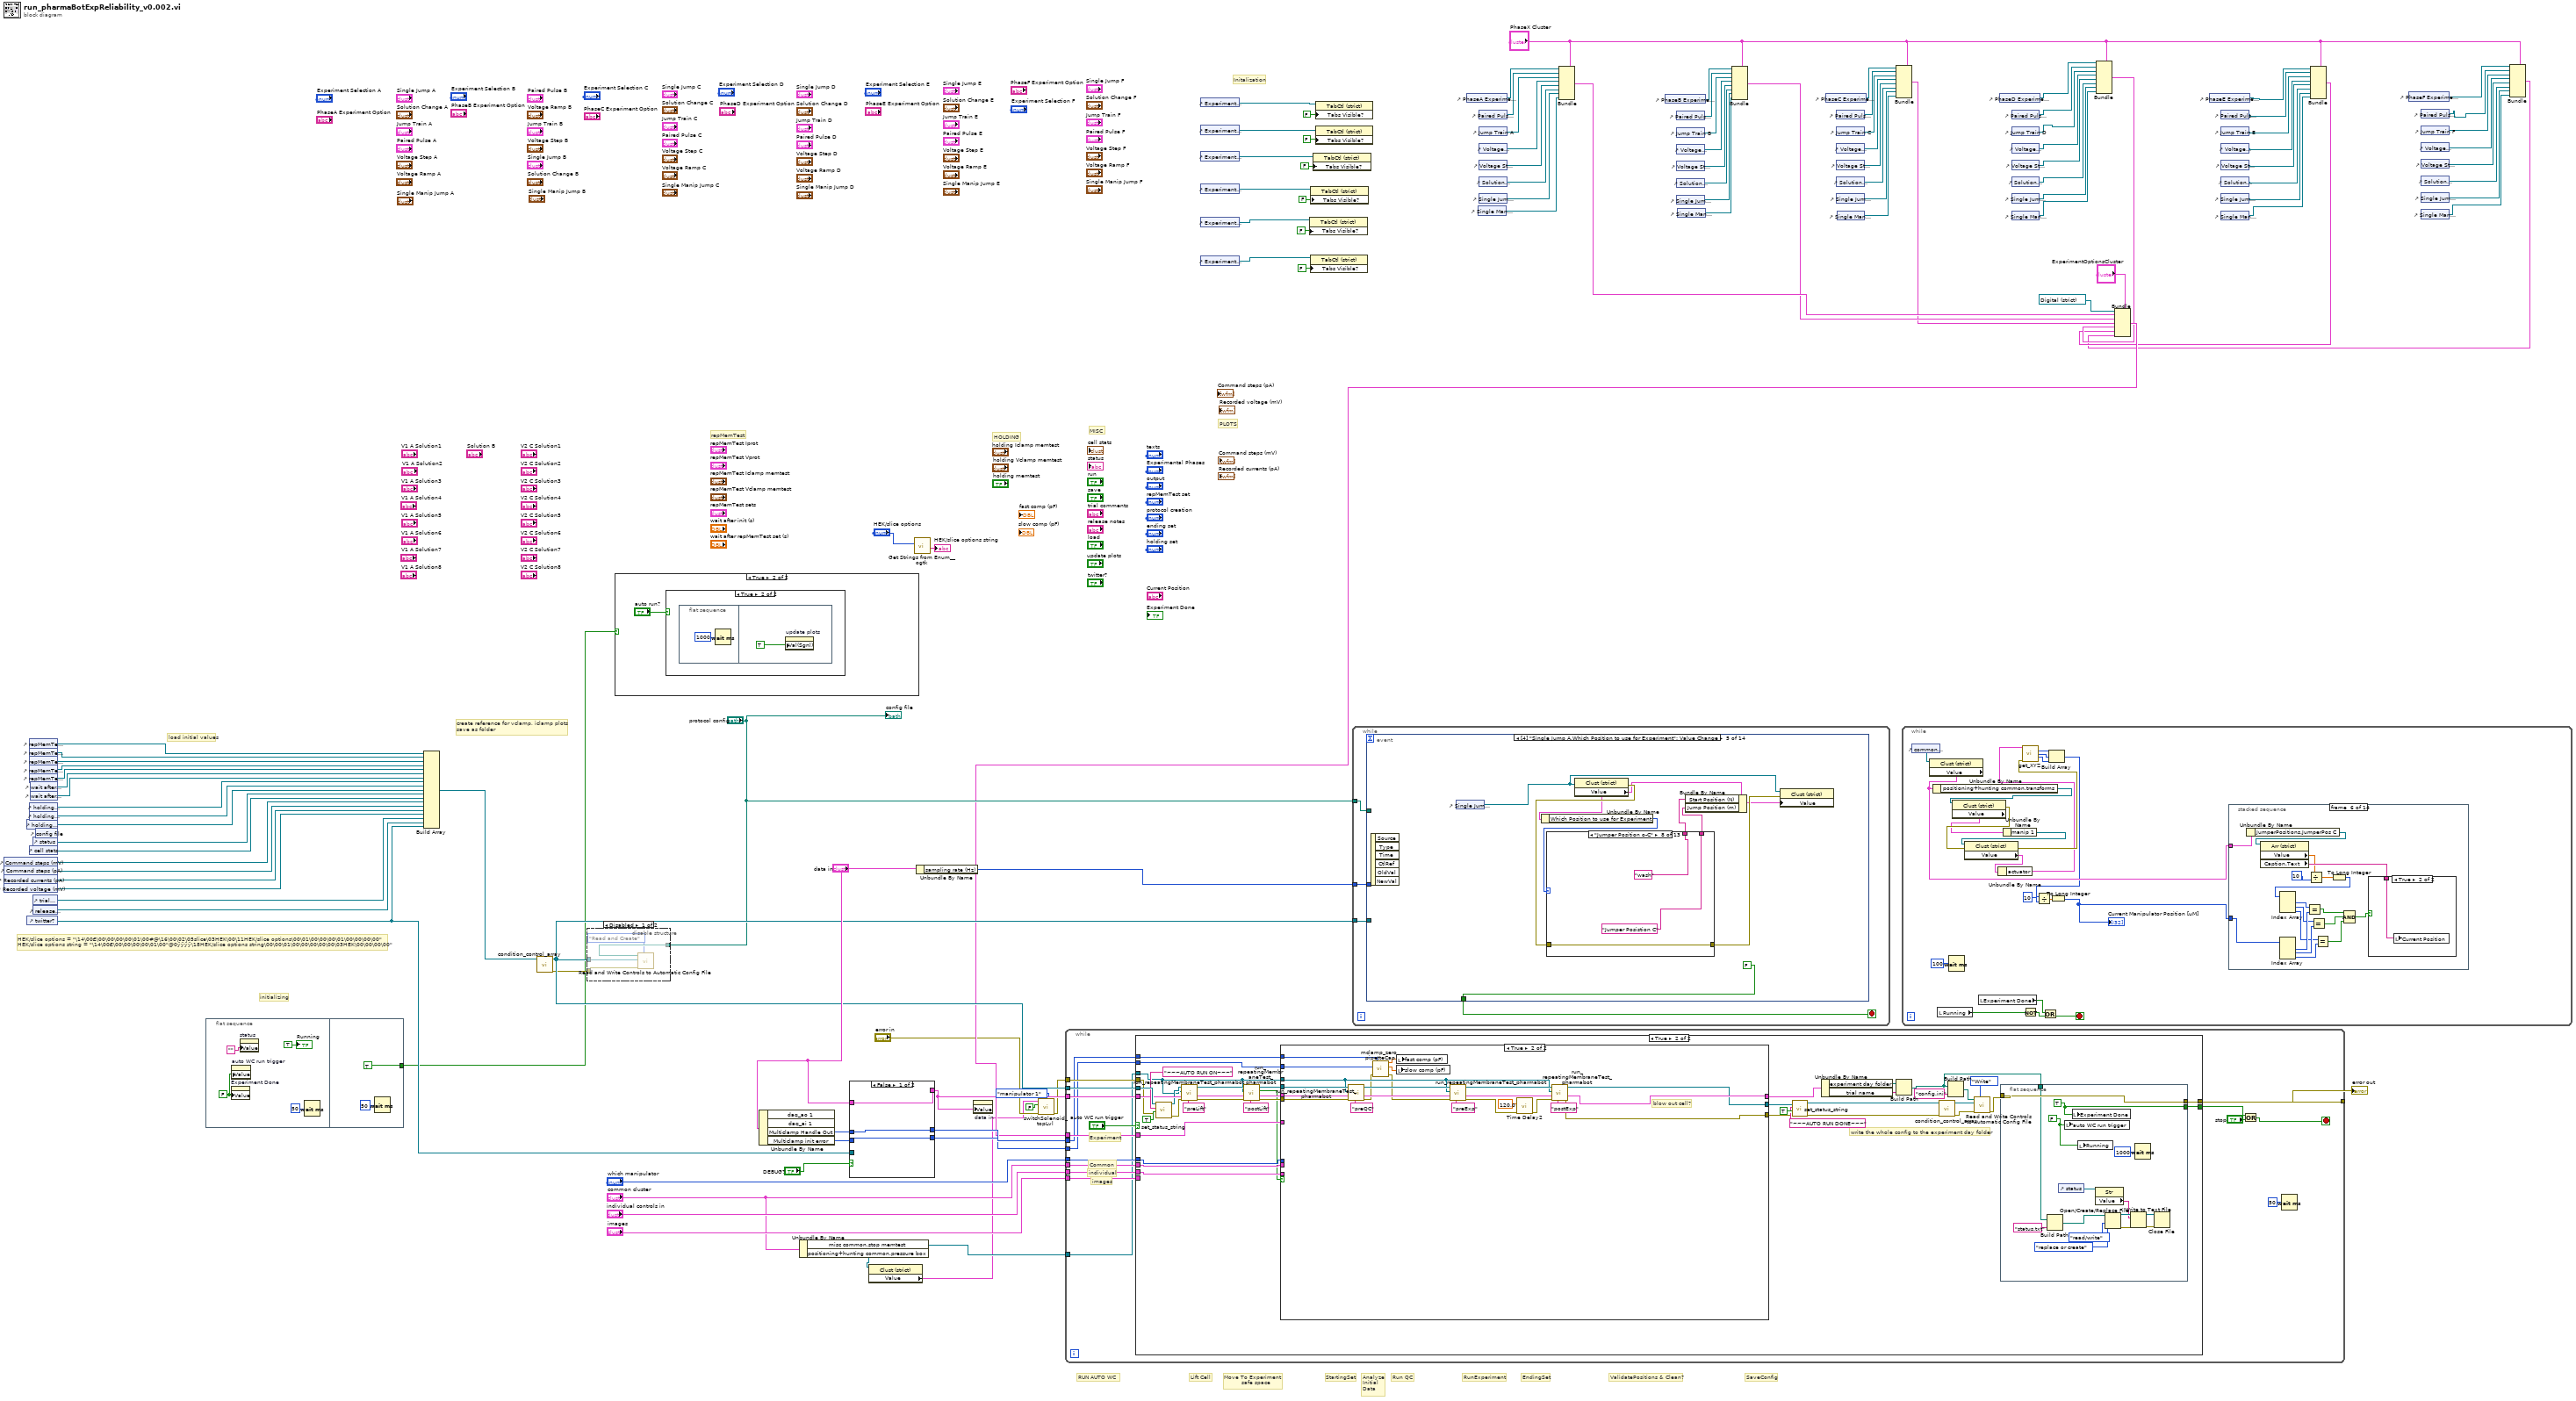
[diagram p0: block diagram]
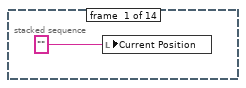
[diagram p3: hidden frame]
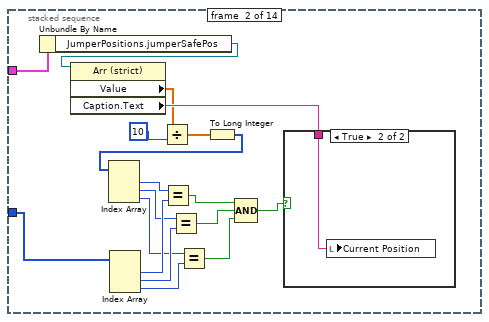
[diagram p4: hidden frame]
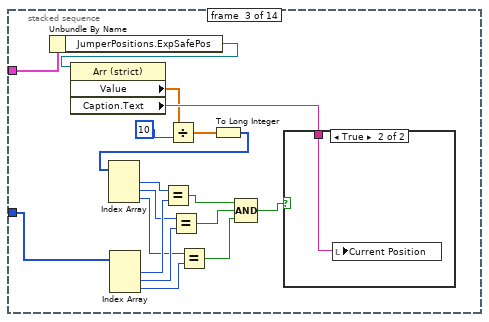
[diagram p6: hidden frame]
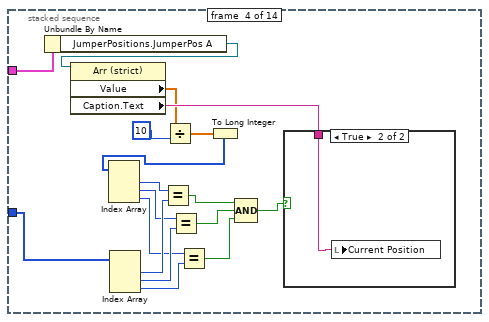
[diagram p8: hidden frame]
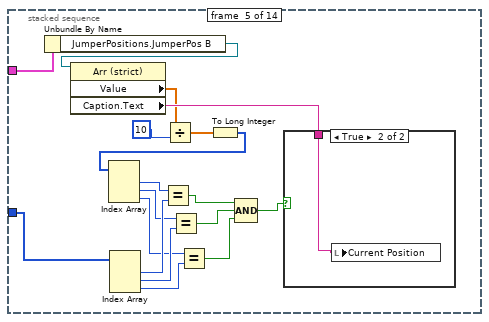
[diagram p10: hidden frame]
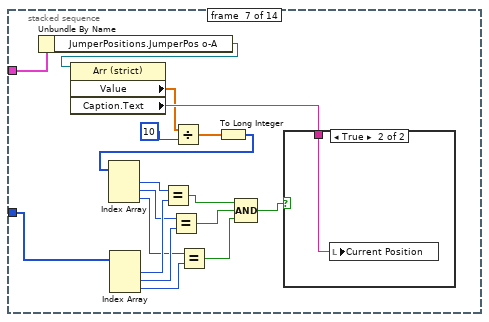
[diagram p13: hidden frame]
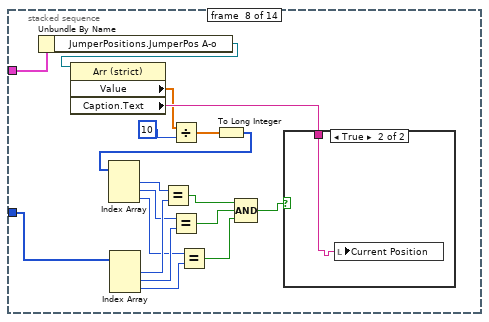
[diagram p15: hidden frame]
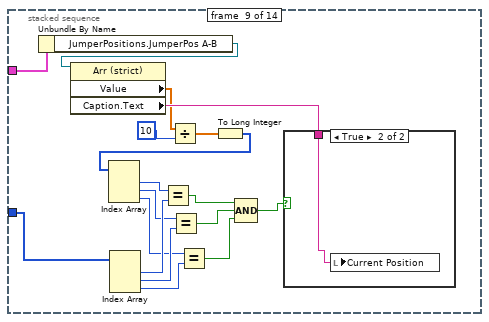
[diagram p17: hidden frame]
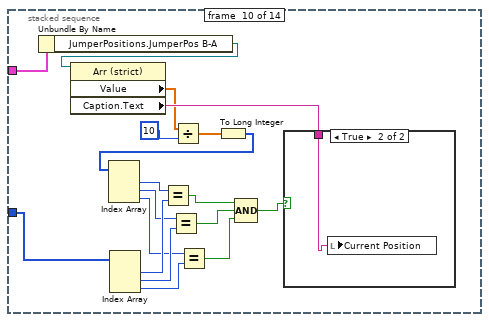
[diagram p19: hidden frame]
diagram:
  # "ValidatePositions & Clean?"
  # "Analyze\nInitial\nData"
  # "SaveConfig"
  # "EndingSet"
  # "RunExperiment"
  # "StartingSet"
  # "Run QC"
  # "Move To Experiment \n          safe space"
  # "Lift Cell"
  # "RUN AUTO WC"
  # "initializing"
  # "Initalization"
  # "HEK/slice options = \"\\14\\00€\\00\\00\\00\\00\\01\\00#@\\16\\00\\02\\05slice\\03HEK\\00\\11HEK/slice options\\00\\01\\00\\00\\00\\01\\00\\00\\00\\00\"\nHEK/slice options string = \"\\14\\00€\\00\\00\\00\\00\\01\\00\"@0ÿÿÿÿ\\18HEK/slice options string\\00\\00\\01\\00\\00\\00\\00\\00\\03HEK\\00\\00\\00\\00\""
  # "PLOTS"
  # "MISC"
  # "create reference for vclamp, iclamp plots\nsave as folder"
  # "load initial values"
  # "HOLDING"
  # "repMemTest"
  n1 = control-ref of="Command steps (mV)"() -> (w83:refnum<vi>)
  n2 = control-ref of="Command steps (pA)"() -> (w89:refnum<vi>)
  n3 = control-ref of="Recorded currents (pA)"() -> (w88:refnum<vi>)
  n4 = control-ref of="Recorded voltage (mV)"() -> (w87:refnum<vi>)
  n5 = control-ref of="holding memtest"() -> (w92:refnum<vi>)
  n6 = control-ref of="twitter?"() -> (w84:refnum<vi>)
  n7 = control-ref of="repMemTest Iprot"() -> (w112:refnum<vi>)
  n8 = control-ref of="repMemTest Vprot"() -> (w111:refnum<vi>)
  n9 = control-ref of="repMemTest Iclamp memtest"() -> (w110:refnum<vi>)
  n10 = control-ref of="repMemTest Vclamp memtest"() -> (w109:refnum<vi>)
  n11 = control-ref of="repMemTest sets"() -> (w113:refnum<vi>)
  n12 = control-ref of="holding Iclamp memtest"() -> (w94:refnum<vi>)
  n13 = control-ref of="holding Vclamp memtest"() -> (w93:refnum<vi>)
  n14 = control-ref of="cell stats"() -> (w90:refnum<vi>)
  n15 = control-ref of="wait after init (s)"() -> (w114:refnum<vi>)
  n16 = control-ref of="wait after repMemTest set (s)"() -> (w115:refnum<vi>)
  n17 = control-ref of="status"() -> (w91:refnum<vi>)
  n18 = control-ref of="trial comments"() -> (w86:refnum<vi>)
  n19 = control-ref of="release notes"() -> (w85:refnum<vi>)
  n20 = control-ref of="config file"() -> ()  [unwired: 1 out]
  n21 = flat-sequence {
    tunnel: [TRUE] -> w45
    frame #0 {
      w119 = FALSE ("Experiment Done")
      n22 = property on="Experiment Done" class="Bool (strict)"("Value"=w119) -> ()  [unwired: 2 in, 2 out]
      n23 = property on="auto WC run trigger" class="Bool (strict)"("Value"=w119) -> ()  [unwired: 2 in, 2 out]
      n24 = property on="status" class="Str"("Value"="") -> ()  [unwired: 2 in, 2 out]
      n25 = Wait (ms)(milliseconds to wait=u32 50) -> ()  [unwired: 1 out]
      "Running" <- TRUE ("Running")
    }
    frame #1 {
      n26 = Wait (ms)(milliseconds to wait=u32 50) -> ()  [unwired: 1 out]
    }
  }
  n27 = Build Array(w112, w111, w110, w109, w113, w114, w115, w94, w93, w92, w91, w90, w83, w89, w88, w87, w86, w85, w84) -> (w101:refnum<vi>[])
  n28 = call "condition_control_array.vi"("control array in"=w101) -> ("error out"=w99:errorcluster, "control array out"=w100:refnum<vi>[])  [unwired: 9 in]
  n29 = disable-structure shown="Disabled" {
    disable-tunnel: w100 -> [w126 _]
    disable-tunnel: w99 -> [w125 _]
    disable-tunnel: "protocol config" -> [w124 _]
    frame Disabled {
      n30 = call "Read and Write Controls to Automatic Config File.vi"("Action"=RWC_Actions."Read and Create", "error in"=w125, "Control References"=w126, "filepath"=w124) -> ()  [unwired: 7 in, 1 out]
    }
    frame Enabled {
    }
  }
  n31 = case shown="True" w45 {
    frame False {
    }
    frame True {
      n32 = case shown="True" "auto run?" {
        frame False {
        }
        frame True {
          n33 = flat-sequence {
            frame #0 {
              n34 = Wait (ms)(milliseconds to wait=u32 1000) -> ()  [unwired: 1 out]
            }
            frame #1 {
              n35 = property on="update plots" class="Bool (strict)"("Val(Sgnl)"=TRUE ("update plots")) -> ()  [unwired: 2 in, 2 out]
            }
          }
        }
      }
    }
  }
  n36 = Unbundle By Name("data in") -> ("Multiclamp Handle Out"=w105:u32, "Multiclamp init error"=w104:i32)  [unwired: 2 out]
  n37 = Unbundle By Name("common cluster") -> ("misc common.stop memtest"=w42:refnum<vi>, "positioning+hunting common.pressure box"=w38:refnum<vi>)
  n38 = case shown="False" "DEBUG?" {
    tunnel: [w132 w138] -> w107
    tunnel: [w131 w137] -> w106
    tunnel: w105 -> [w132 _]
    tunnel: w104 -> [w131 _]
    tunnel: "data in" -> [w130 w136]
    tunnel: [w130 w135] -> w102
    tunnel: w84 -> [_ w134]
    frame False {
    }
    frame True {
      n39 = call "init multiclamp.vi"() -> ("Error out"=w137:i32, "Multiclamp Handle Out"=w138:u32)  [unwired: 9 in, 1 out]
      n40 = Bundle By Name(cluster=w136, "Multiclamp Handle Out"=w138, "Multiclamp init error"=w137) -> (w135:T9)
      n41 = property class="Bool (strict)"(reference=w134, "Value"=FALSE) -> ()  [unwired: 1 in, 2 out]
    }
  }
  n42 = property class="Clust (strict)"(reference=w38) -> ("Value"=w37:T26)  [unwired: 1 in, 2 out]
  n43 = call "Get Strings from Enum__ogtk.vi"("Enum"="HEK/slice options") -> ("String Value"=→"HEK/slice options string":string)  [unwired: 7 in, 3 out]
  n44 = Unbundle By Name("data in") -> ("sampling rate (Hz)"=w116:i32)
  n45 = property on="data in" class="Clust (strict)"("Value"=w102) -> ()  [unwired: 2 in, 2 out]
  n46 = call "switchSolenoid_topLvl.vi"("which manipulator"=T10."manipulator 1", "error in (no error)"="error in", "solenoidSwitch (T:atm; F: Reg)"=FALSE, "Pressure box control in"=w37) -> ("error out"=w39:errorcluster)  [unwired: 6 in, 1 out]
  n47 = control-ref of="Experiment Selection A"() -> (w81:refnum<vi>)
  n48 = control-ref of="Experiment Selection B"() -> (w78:refnum<vi>)
  n49 = control-ref of="Experiment Selection C"() -> (w58:refnum<vi>)
  n50 = control-ref of="Experiment Selection D"() -> (w4:refnum<vi>)
  n51 = control-ref of="Experiment Selection E"() -> (w3:refnum<vi>)
  n52 = control-ref of="Experiment Selection F"() -> (w2:refnum<vi>)
  n53 = property class="TabCtl (strict)"(reference=w3, "Tabs Visible?"=FALSE) -> ()  [unwired: 1 in, 2 out]
  n54 = property class="TabCtl (strict)"(reference=w2, "Tabs Visible?"=FALSE) -> ()  [unwired: 1 in, 2 out]
  n55 = property class="TabCtl (strict)"(reference=w4, "Tabs Visible?"=FALSE) -> ()  [unwired: 1 in, 2 out]
  n56 = property class="TabCtl (strict)"(reference=w58, "Tabs Visible?"=FALSE) -> ()  [unwired: 1 in, 2 out]
  n57 = property class="TabCtl (strict)"(reference=w81, "Tabs Visible?"=FALSE) -> ()  [unwired: 1 in, 2 out]
  n58 = property class="TabCtl (strict)"(reference=w78, "Tabs Visible?"=FALSE) -> ()  [unwired: 1 in, 2 out]
  n59 = while {
    tunnel: w116 -> [w142]
    tunnel: "protocol config" -> [w141]
    tunnel: w100 -> [w140]
    stop <- w139 stop-if-true
    n60 = event shown="[4] \"Single Jump A.Which Position to use for Experiment\": Value Change" {
      selector: _ -> [_ _ _ _ _ _ _ _ _ _ _ _ _ _]
      dyn-events: _ -> [_ _ _ _ _ _ _ _ _ _ _ _ _ _]
      timeout: _ -> [_ _ _ _ _ _ _ _ _ _ _ _ _ _]
      tunnel: w142 -> [_ _ _ _ _ _ _ _ _ _ w619 _ _ _]
      tunnel: w141 -> [_ _ _ _ _ _ _ _ _ _ _ _ w666 _]
      tunnel: w140 -> [_ _ _ _ _ _ _ _ _ _ _ _ w665 w683]
      tunnel: [w143 w161 _ FALSE ("NewVal") FALSE ("NewVal") FALSE ("NewVal") FALSE ("NewVal") FALSE ("NewVal") FALSE ("NewVal") FALSE ("NewVal") w618 TRUE ("NewVal") FALSE ("NewVal") FALSE ("NewVal")] -> w139
      event Timeout {
        n61 = event-data() -> ()  [unwired: 1 in, 3 out]
        n62 = local read "Running"() -> (w144:bool)
        n63 = case shown="False" w144 {
          tunnel: [w146 FALSE] -> w143
          frame False {
            n64 = local read "Experiment Done"() -> (w146:bool)
          }
          frame True {
          }
        }
        n65 = Wait (ms)(milliseconds to wait=u32 50) -> ()  [unwired: 1 out]
      }
      event "stop": Value Change {
        n66 = event-data() -> ("NewVal"=w161:bool)  [unwired: 1 in, 5 out]
        n67 = Not(x=w161) -> (.not. x?=w160:bool)
        n68 = property on="Experiment Done" class="Bool (strict)"("Value"=w161) -> ()  [unwired: 2 in, 2 out]
        n69 = property on="Running" class="Bool (strict)"("Value"=w160) -> ()  [unwired: 2 in, 2 out]
        n70 = control-ref of="Experiment Selection A"() -> (w159:refnum<vi>)
        n71 = control-ref of="Experiment Selection B"() -> (w156:refnum<vi>)
        n72 = control-ref of="Experiment Selection C"() -> (w155:refnum<vi>)
        n73 = control-ref of="Experiment Selection D"() -> (w150:refnum<vi>)
        n74 = control-ref of="Experiment Selection E"() -> (w149:refnum<vi>)
        n75 = control-ref of="Experiment Selection F"() -> (w148:refnum<vi>)
        n76 = property class="TabCtl (strict)"(reference=w149, "Tabs Visible?"=TRUE) -> ()  [unwired: 1 in, 2 out]
        n77 = property class="TabCtl (strict)"(reference=w148, "Tabs Visible?"=TRUE) -> ()  [unwired: 1 in, 2 out]
        n78 = property class="TabCtl (strict)"(reference=w150, "Tabs Visible?"=TRUE) -> ()  [unwired: 1 in, 2 out]
        n79 = property class="TabCtl (strict)"(reference=w155, "Tabs Visible?"=TRUE) -> ()  [unwired: 1 in, 2 out]
        n80 = property class="TabCtl (strict)"(reference=w159, "Tabs Visible?"=TRUE) -> ()  [unwired: 1 in, 2 out]
        n81 = property class="TabCtl (strict)"(reference=w156, "Tabs Visible?"=TRUE) -> ()  [unwired: 1 in, 2 out]
        n82 = Wait (ms)(milliseconds to wait=u32 1000) -> ()  [unwired: 1 out]
      }
      event "Experiment Done": Value Change {
        n83 = event-data() -> ()  [unwired: 1 in, 6 out]
        n84 = control-ref of="Experiment Selection A"() -> (w175:refnum<vi>)
        n85 = control-ref of="Experiment Selection B"() -> (w172:refnum<vi>)
        n86 = control-ref of="Experiment Selection C"() -> (w171:refnum<vi>)
        n87 = control-ref of="Experiment Selection D"() -> (w166:refnum<vi>)
        n88 = control-ref of="Experiment Selection E"() -> (w165:refnum<vi>)
        n89 = control-ref of="Experiment Selection F"() -> (w164:refnum<vi>)
        n90 = property class="TabCtl (strict)"(reference=w165, "Tabs Visible?"=TRUE) -> ()  [unwired: 1 in, 2 out]
        n91 = property class="TabCtl (strict)"(reference=w164, "Tabs Visible?"=TRUE) -> ()  [unwired: 1 in, 2 out]
        n92 = property class="TabCtl (strict)"(reference=w166, "Tabs Visible?"=TRUE) -> ()  [unwired: 1 in, 2 out]
        n93 = property class="TabCtl (strict)"(reference=w171, "Tabs Visible?"=TRUE) -> ()  [unwired: 1 in, 2 out]
        n94 = property class="TabCtl (strict)"(reference=w175, "Tabs Visible?"=TRUE) -> ()  [unwired: 1 in, 2 out]
        n95 = property class="TabCtl (strict)"(reference=w172, "Tabs Visible?"=TRUE) -> ()  [unwired: 1 in, 2 out]
        n96 = Wait (ms)(milliseconds to wait=u32 100) -> ()  [unwired: 1 out]
      }
      event "PhaseA Experiment Option", "PhaseB Experiment Option", "PhaseC Experiment Option", "PhaseD Experiment Option", "PhaseE Experiment Option", "PhaseF Experiment Option": Value Change {
        n97 = event-data() -> ("CtlRef"=w177:refnum<vi>, "NewVal"=w176:string)  [unwired: 1 in, 4 out]
        n98 = property class="CmbBox"(reference=w177) -> ("Label.Text"=w179:string)  [unwired: 1 in, 2 out]
        n99 = case shown="\"PhaseF Experiment Option\"" w179 {
          tunnel: w176 -> [_ w181 w206 w231 w256 w281 w306]
          frame "Null", Default {
          }
          frame "PhaseA Experiment Option" {
            n100 = control-ref of="Experiment Selection A"() -> (w180:refnum<vi>)
            n101 = case shown="\"Single Manip Jump\"" w181 {
              tunnel: w180 -> [_ w183 w186 w189 w192 w195 w198 w201 w203]
              frame "False", Default {
              }
              frame "Single Jump" {
                n102 = property class="TabCtl (strict)"(reference=w183, "Value"=T17."Single Jump" ("Experiment Selection A")) -> ()  [unwired: 1 in, 2 out]
                n103 = property class="TabCtl (strict)"(reference=w183, "Visible"=TRUE) -> ()  [unwired: 1 in, 2 out]
              }
              frame "Solution Change" {
                n104 = property class="TabCtl (strict)"(reference=w186, "Visible"=TRUE) -> ()  [unwired: 1 in, 2 out]
                n105 = property class="TabCtl (strict)"(reference=w186, "Value"=T17."Solution Change" ("Experiment Selection A")) -> ()  [unwired: 1 in, 2 out]
              }
              frame "Voltage Step" {
                n106 = property class="TabCtl (strict)"(reference=w189, "Value"=T17."Voltage Step" ("Experiment Selection A")) -> ()  [unwired: 1 in, 2 out]
                n107 = property class="TabCtl (strict)"(reference=w189, "Visible"=TRUE) -> ()  [unwired: 1 in, 2 out]
              }
              frame "Voltage Ramp" {
                n108 = property class="TabCtl (strict)"(reference=w192, "Value"=T17."Voltage Ramp" ("Experiment Selection A")) -> ()  [unwired: 1 in, 2 out]
                n109 = property class="TabCtl (strict)"(reference=w192, "Visible"=TRUE) -> ()  [unwired: 1 in, 2 out]
              }
              frame "Jump Train" {
                n110 = property class="TabCtl (strict)"(reference=w195, "Value"=T17."Jump Train" ("Experiment Selection A")) -> ()  [unwired: 1 in, 2 out]
                n111 = property class="TabCtl (strict)"(reference=w195, "Visible"=TRUE) -> ()  [unwired: 1 in, 2 out]
              }
              frame "Paired Pulse" {
                n112 = property class="TabCtl (strict)"(reference=w198, "Value"=T17."Paired Pulse" ("Experiment Selection A")) -> ()  [unwired: 1 in, 2 out]
                n113 = property class="TabCtl (strict)"(reference=w198, "Visible"=TRUE) -> ()  [unwired: 1 in, 2 out]
              }
              frame "Single Manip Jump" {
                n114 = property class="TabCtl (strict)"(reference=w201, "Value"=T17."Single Manip Jump" ("Experiment Selection A")) -> ()  [unwired: 1 in, 2 out]
                n115 = property class="TabCtl (strict)"(reference=w201, "Visible"=TRUE) -> ()  [unwired: 1 in, 2 out]
              }
              frame "none" {
                n116 = property class="TabCtl (strict)"(reference=w203, "Visible"=FALSE) -> ()  [unwired: 1 in, 2 out]
              }
            }
          }
          frame "PhaseC Experiment Option" {
            n117 = control-ref of="Experiment Selection C"() -> (w205:refnum<vi>)
            n118 = case shown="\"Single Manip Jump\"" w206 {
              tunnel: w205 -> [_ w208 w211 w214 w217 w220 w223 w226 w228]
              frame "False", Default {
              }
              frame "Single Jump" {
                n119 = property class="TabCtl (strict)"(reference=w208, "Value"=T17."Single Jump" ("Experiment Selection A")) -> ()  [unwired: 1 in, 2 out]
                n120 = property class="TabCtl (strict)"(reference=w208, "Visible"=TRUE) -> ()  [unwired: 1 in, 2 out]
              }
              frame "Solution Change" {
                n121 = property class="TabCtl (strict)"(reference=w211, "Visible"=TRUE) -> ()  [unwired: 1 in, 2 out]
                n122 = property class="TabCtl (strict)"(reference=w211, "Value"=T17."Solution Change" ("Experiment Selection A")) -> ()  [unwired: 1 in, 2 out]
              }
              frame "Voltage Step" {
                n123 = property class="TabCtl (strict)"(reference=w214, "Value"=T17."Voltage Step" ("Experiment Selection A")) -> ()  [unwired: 1 in, 2 out]
                n124 = property class="TabCtl (strict)"(reference=w214, "Visible"=TRUE) -> ()  [unwired: 1 in, 2 out]
              }
              frame "Voltage Ramp" {
                n125 = property class="TabCtl (strict)"(reference=w217, "Value"=T17."Voltage Ramp" ("Experiment Selection A")) -> ()  [unwired: 1 in, 2 out]
                n126 = property class="TabCtl (strict)"(reference=w217, "Visible"=TRUE) -> ()  [unwired: 1 in, 2 out]
              }
              frame "Jump Train" {
                n127 = property class="TabCtl (strict)"(reference=w220, "Value"=T17."Jump Train" ("Experiment Selection A")) -> ()  [unwired: 1 in, 2 out]
                n128 = property class="TabCtl (strict)"(reference=w220, "Visible"=TRUE) -> ()  [unwired: 1 in, 2 out]
              }
              frame "Paired Pulse" {
                n129 = property class="TabCtl (strict)"(reference=w223, "Value"=T17."Paired Pulse" ("Experiment Selection A")) -> ()  [unwired: 1 in, 2 out]
                n130 = property class="TabCtl (strict)"(reference=w223, "Visible"=TRUE) -> ()  [unwired: 1 in, 2 out]
              }
              frame "Single Manip Jump" {
                n131 = property class="TabCtl (strict)"(reference=w226, "Value"=T17."Single Manip Jump" ("Experiment Selection A")) -> ()  [unwired: 1 in, 2 out]
                n132 = property class="TabCtl (strict)"(reference=w226, "Visible"=TRUE) -> ()  [unwired: 1 in, 2 out]
              }
              frame "none" {
                n133 = property class="TabCtl (strict)"(reference=w228, "Visible"=FALSE) -> ()  [unwired: 1 in, 2 out]
              }
            }
          }
          frame "PhaseB Experiment Option" {
            n134 = control-ref of="Experiment Selection B"() -> (w230:refnum<vi>)
            n135 = case shown="\"Single Manip Jump\"" w231 {
              tunnel: w230 -> [_ w233 w236 w239 w242 w245 w248 w251 w253]
              frame "False", Default {
              }
              frame "Single Jump" {
                n136 = property class="TabCtl (strict)"(reference=w233, "Value"=T17."Single Jump" ("Experiment Selection A")) -> ()  [unwired: 1 in, 2 out]
                n137 = property class="TabCtl (strict)"(reference=w233, "Visible"=TRUE) -> ()  [unwired: 1 in, 2 out]
              }
              frame "Solution Change" {
                n138 = property class="TabCtl (strict)"(reference=w236, "Visible"=TRUE) -> ()  [unwired: 1 in, 2 out]
                n139 = property class="TabCtl (strict)"(reference=w236, "Value"=T17."Solution Change" ("Experiment Selection A")) -> ()  [unwired: 1 in, 2 out]
              }
              frame "Voltage Step" {
                n140 = property class="TabCtl (strict)"(reference=w239, "Value"=T17."Voltage Step" ("Experiment Selection A")) -> ()  [unwired: 1 in, 2 out]
                n141 = property class="TabCtl (strict)"(reference=w239, "Visible"=TRUE) -> ()  [unwired: 1 in, 2 out]
              }
              frame "Voltage Ramp" {
                n142 = property class="TabCtl (strict)"(reference=w242, "Value"=T17."Voltage Ramp" ("Experiment Selection A")) -> ()  [unwired: 1 in, 2 out]
                n143 = property class="TabCtl (strict)"(reference=w242, "Visible"=TRUE) -> ()  [unwired: 1 in, 2 out]
              }
              frame "Jump Train" {
                n144 = property class="TabCtl (strict)"(reference=w245, "Value"=T17."Jump Train" ("Experiment Selection A")) -> ()  [unwired: 1 in, 2 out]
                n145 = property class="TabCtl (strict)"(reference=w245, "Visible"=TRUE) -> ()  [unwired: 1 in, 2 out]
              }
              frame "Paired Pulse" {
                n146 = property class="TabCtl (strict)"(reference=w248, "Value"=T17."Paired Pulse" ("Experiment Selection A")) -> ()  [unwired: 1 in, 2 out]
                n147 = property class="TabCtl (strict)"(reference=w248, "Visible"=TRUE) -> ()  [unwired: 1 in, 2 out]
              }
              frame "Single Manip Jump" {
                n148 = property class="TabCtl (strict)"(reference=w251, "Value"=T17."Single Manip Jump" ("Experiment Selection A")) -> ()  [unwired: 1 in, 2 out]
                n149 = property class="TabCtl (strict)"(reference=w251, "Visible"=TRUE) -> ()  [unwired: 1 in, 2 out]
              }
              frame "none" {
                n150 = property class="TabCtl (strict)"(reference=w253, "Visible"=FALSE) -> ()  [unwired: 1 in, 2 out]
              }
            }
          }
          frame "PhaseD Experiment Option" {
            n151 = control-ref of="Experiment Selection D"() -> (w255:refnum<vi>)
            n152 = case shown="\"Single Manip Jump\"" w256 {
              tunnel: w255 -> [_ w258 w261 w264 w267 w270 w273 w276 w278]
              frame "False", Default {
              }
              frame "Single Jump" {
                n153 = property class="TabCtl (strict)"(reference=w258, "Value"=T17."Single Jump" ("Experiment Selection A")) -> ()  [unwired: 1 in, 2 out]
                n154 = property class="TabCtl (strict)"(reference=w258, "Visible"=TRUE) -> ()  [unwired: 1 in, 2 out]
              }
              frame "Solution Change" {
                n155 = property class="TabCtl (strict)"(reference=w261, "Visible"=TRUE) -> ()  [unwired: 1 in, 2 out]
                n156 = property class="TabCtl (strict)"(reference=w261, "Value"=T17."Solution Change" ("Experiment Selection A")) -> ()  [unwired: 1 in, 2 out]
              }
              frame "Voltage Step" {
                n157 = property class="TabCtl (strict)"(reference=w264, "Value"=T17."Voltage Step" ("Experiment Selection A")) -> ()  [unwired: 1 in, 2 out]
                n158 = property class="TabCtl (strict)"(reference=w264, "Visible"=TRUE) -> ()  [unwired: 1 in, 2 out]
              }
              frame "Voltage Ramp" {
                n159 = property class="TabCtl (strict)"(reference=w267, "Value"=T17."Voltage Ramp" ("Experiment Selection A")) -> ()  [unwired: 1 in, 2 out]
                n160 = property class="TabCtl (strict)"(reference=w267, "Visible"=TRUE) -> ()  [unwired: 1 in, 2 out]
              }
              frame "Jump Train" {
                n161 = property class="TabCtl (strict)"(reference=w270, "Value"=T17."Jump Train" ("Experiment Selection A")) -> ()  [unwired: 1 in, 2 out]
                n162 = property class="TabCtl (strict)"(reference=w270, "Visible"=TRUE) -> ()  [unwired: 1 in, 2 out]
              }
              frame "Paired Pulse" {
                n163 = property class="TabCtl (strict)"(reference=w273, "Value"=T17."Paired Pulse" ("Experiment Selection A")) -> ()  [unwired: 1 in, 2 out]
                n164 = property class="TabCtl (strict)"(reference=w273, "Visible"=TRUE) -> ()  [unwired: 1 in, 2 out]
              }
              frame "Single Manip Jump" {
                n165 = property class="TabCtl (strict)"(reference=w276, "Value"=T17."Single Manip Jump" ("Experiment Selection A")) -> ()  [unwired: 1 in, 2 out]
                n166 = property class="TabCtl (strict)"(reference=w276, "Visible"=TRUE) -> ()  [unwired: 1 in, 2 out]
              }
              frame "none" {
                n167 = property class="TabCtl (strict)"(reference=w278, "Visible"=FALSE) -> ()  [unwired: 1 in, 2 out]
              }
            }
          }
          frame "PhaseE Experiment Option" {
            n168 = control-ref of="Experiment Selection E"() -> (w280:refnum<vi>)
            n169 = case shown="\"Single Manip Jump\"" w281 {
              tunnel: w280 -> [_ w283 w286 w289 w292 w295 w298 w301 w303]
              frame "False", Default {
              }
              frame "Single Jump" {
                n170 = property class="TabCtl (strict)"(reference=w283, "Value"=T17."Single Jump" ("Experiment Selection A")) -> ()  [unwired: 1 in, 2 out]
                n171 = property class="TabCtl (strict)"(reference=w283, "Visible"=TRUE) -> ()  [unwired: 1 in, 2 out]
              }
              frame "Solution Change" {
                n172 = property class="TabCtl (strict)"(reference=w286, "Visible"=TRUE) -> ()  [unwired: 1 in, 2 out]
                n173 = property class="TabCtl (strict)"(reference=w286, "Value"=T17."Solution Change" ("Experiment Selection A")) -> ()  [unwired: 1 in, 2 out]
              }
              frame "Voltage Step" {
                n174 = property class="TabCtl (strict)"(reference=w289, "Value"=T17."Voltage Step" ("Experiment Selection A")) -> ()  [unwired: 1 in, 2 out]
                n175 = property class="TabCtl (strict)"(reference=w289, "Visible"=TRUE) -> ()  [unwired: 1 in, 2 out]
              }
              frame "Voltage Ramp" {
                n176 = property class="TabCtl (strict)"(reference=w292, "Value"=T17."Voltage Ramp" ("Experiment Selection A")) -> ()  [unwired: 1 in, 2 out]
                n177 = property class="TabCtl (strict)"(reference=w292, "Visible"=TRUE) -> ()  [unwired: 1 in, 2 out]
              }
              frame "Jump Train" {
                n178 = property class="TabCtl (strict)"(reference=w295, "Value"=T17."Jump Train" ("Experiment Selection A")) -> ()  [unwired: 1 in, 2 out]
                n179 = property class="TabCtl (strict)"(reference=w295, "Visible"=TRUE) -> ()  [unwired: 1 in, 2 out]
              }
              frame "Paired Pulse" {
                n180 = property class="TabCtl (strict)"(reference=w298, "Value"=T17."Paired Pulse" ("Experiment Selection A")) -> ()  [unwired: 1 in, 2 out]
                n181 = property class="TabCtl (strict)"(reference=w298, "Visible"=TRUE) -> ()  [unwired: 1 in, 2 out]
              }
              frame "Single Manip Jump" {
                n182 = property class="TabCtl (strict)"(reference=w301, "Value"=T17."Single Manip Jump" ("Experiment Selection A")) -> ()  [unwired: 1 in, 2 out]
                n183 = property class="TabCtl (strict)"(reference=w301, "Visible"=TRUE) -> ()  [unwired: 1 in, 2 out]
              }
              frame "none" {
                n184 = property class="TabCtl (strict)"(reference=w303, "Visible"=FALSE) -> ()  [unwired: 1 in, 2 out]
              }
            }
          }
          frame "PhaseF Experiment Option" {
            n185 = control-ref of="Experiment Selection F"() -> (w305:refnum<vi>)
            n186 = case shown="\"Single Manip Jump\"" w306 {
              tunnel: w305 -> [_ w308 w311 w314 w317 w320 w323 w326 w328]
              frame "False", Default {
              }
              frame "Single Jump" {
                n187 = property class="TabCtl (strict)"(reference=w308, "Value"=T17."Single Jump" ("Experiment Selection A")) -> ()  [unwired: 1 in, 2 out]
                n188 = property class="TabCtl (strict)"(reference=w308, "Visible"=TRUE) -> ()  [unwired: 1 in, 2 out]
              }
              frame "Solution Change" {
                n189 = property class="TabCtl (strict)"(reference=w311, "Visible"=TRUE) -> ()  [unwired: 1 in, 2 out]
                n190 = property class="TabCtl (strict)"(reference=w311, "Value"=T17."Solution Change" ("Experiment Selection A")) -> ()  [unwired: 1 in, 2 out]
              }
              frame "Voltage Step" {
                n191 = property class="TabCtl (strict)"(reference=w314, "Value"=T17."Voltage Step" ("Experiment Selection A")) -> ()  [unwired: 1 in, 2 out]
                n192 = property class="TabCtl (strict)"(reference=w314, "Visible"=TRUE) -> ()  [unwired: 1 in, 2 out]
              }
              frame "Voltage Ramp" {
                n193 = property class="TabCtl (strict)"(reference=w317, "Value"=T17."Voltage Ramp" ("Experiment Selection A")) -> ()  [unwired: 1 in, 2 out]
                n194 = property class="TabCtl (strict)"(reference=w317, "Visible"=TRUE) -> ()  [unwired: 1 in, 2 out]
              }
              frame "Jump Train" {
                n195 = property class="TabCtl (strict)"(reference=w320, "Value"=T17."Jump Train" ("Experiment Selection A")) -> ()  [unwired: 1 in, 2 out]
                n196 = property class="TabCtl (strict)"(reference=w320, "Visible"=TRUE) -> ()  [unwired: 1 in, 2 out]
              }
              frame "Paired Pulse" {
                n197 = property class="TabCtl (strict)"(reference=w323, "Value"=T17."Paired Pulse" ("Experiment Selection A")) -> ()  [unwired: 1 in, 2 out]
                n198 = property class="TabCtl (strict)"(reference=w323, "Visible"=TRUE) -> ()  [unwired: 1 in, 2 out]
              }
              frame "Single Manip Jump" {
                n199 = property class="TabCtl (strict)"(reference=w326, "Value"=T17."Single Manip Jump" ("Experiment Selection A")) -> ()  [unwired: 1 in, 2 out]
                n200 = property class="TabCtl (strict)"(reference=w326, "Visible"=TRUE) -> ()  [unwired: 1 in, 2 out]
              }
              frame "none" {
                n201 = property class="TabCtl (strict)"(reference=w328, "Visible"=FALSE) -> ()  [unwired: 1 in, 2 out]
              }
            }
          }
        }
      }
      event "Single Jump A.Which Position to use for Experiment": Value Change {
        n202 = event-data() -> ()  [unwired: 1 in, 6 out]
        n203 = control-ref of="Single Jump A"() -> (w333:refnum<vi>)
        n204 = property class="Clust (strict)"(reference=w333) -> (error out=w337:errorcluster, "Value"=w332:T18)  [unwired: 1 in, 1 out]
        n205 = Unbundle By Name(w332) -> ("Which Position to use for Experiment"=w331:T28)
        n206 = case shown="\"Jumper Position o-C\"" w331 {
          tunnel: ["Experiment Safe Posistion" "Jumper Posistion A" "Jumper Posistion B" "Jumper Posistion B" "Jumper Posistion C" "wash" "Jumper Posistion C" "wash" "Jumper Posistion A" "Jumper Posistion A" "Jumper Safe Posistion" "Jumper Posistion B" "Jumper Posistion C"] -> w335
          tunnel: ["NA" "Jumper Posistion B" "Jumper Posistion A" "Jumper Posistion C" "Jumper Posistion B" "Jumper Posistion A" "wash" "Jumper Posistion C" "wash" "NA" "NA" "NA" "NA"] -> w336
          tunnel: w337 -> [w340 w344 w347 w350 w353 w355 w358 w361 w364 w367 w370 w373 w376]
          tunnel: [w340 w344 w347 w350 w353 w355 w358 w361 w364 w367 w370 w373 w376] -> w338
          frame "Experiment Safe Position" {
          }
          frame "Jumper Position A-B" {
          }
          frame "Jumper Position B-A" {
          }
          frame "Jumper Position B-C" {
          }
          frame "Jumper Position C-B" {
          }
          frame "Jumper Position o-A" {
          }
          frame "Jumper Position C-o" {
          }
          frame "Jumper Position o-C" {
          }
          frame "Jumper Position A-o" {
          }
          frame "Jumper Position A" {
          }
          frame "Jumper Safe Position" {
          }
          frame "Jumper Position B" {
          }
          frame "Jumper Position C" {
          }
        }
        n207 = Bundle By Name(cluster=w332, "Start Position (N)"=w335, "Jump Position (m)"=w336) -> (w334:T18)
        n208 = property class="Clust (strict)"(reference=w333, error in=w338, "Value"=w334) -> ()  [unwired: 2 out]
      }
      event "Single Jump B.Which Position to use for Experiment": Value Change {
        n209 = event-data() -> ()  [unwired: 1 in, 6 out]
        n210 = control-ref of="Single Jump B"() -> (w381:refnum<vi>)
        n211 = property class="Clust (strict)"(reference=w381) -> (error out=w385:errorcluster, "Value"=w380:T18)  [unwired: 1 in, 1 out]
        n212 = Unbundle By Name(w380) -> ("Which Position to use for Experiment"=w379:T28)
        n213 = case shown="\"Jumper Position o-C\"" w379 {
          tunnel: ["Experiment Safe Posistion" "Jumper Posistion A" "Jumper Posistion B" "Jumper Posistion B" "Jumper Posistion C" "wash" "Jumper Posistion C" "wash" "Jumper Posistion A" "Jumper Posistion A" "Jumper Safe Posistion" "Jumper Posistion B" "Jumper Posistion C"] -> w383
          tunnel: ["NA" "Jumper Posistion B" "Jumper Posistion A" "Jumper Posistion C" "Jumper Posistion B" "Jumper Posistion A" "wash" "Jumper Posistion C" "wash" "NA" "NA" "NA" "NA"] -> w384
          tunnel: w385 -> [w388 w392 w395 w398 w401 w403 w406 w409 w412 w415 w418 w421 w424]
          tunnel: [w388 w392 w395 w398 w401 w403 w406 w409 w412 w415 w418 w421 w424] -> w386
          frame "Experiment Safe Position" {
          }
          frame "Jumper Position A-B" {
          }
          frame "Jumper Position B-A" {
          }
          frame "Jumper Position B-C" {
          }
          frame "Jumper Position C-B" {
          }
          frame "Jumper Position o-A" {
          }
          frame "Jumper Position C-o" {
          }
          frame "Jumper Position o-C" {
          }
          frame "Jumper Position A-o" {
          }
          frame "Jumper Position A" {
          }
          frame "Jumper Safe Position" {
          }
          frame "Jumper Position B" {
          }
          frame "Jumper Position C" {
          }
        }
        n214 = Bundle By Name(cluster=w380, "Start Position (N)"=w383, "Jump Position (m)"=w384) -> (w382:T18)
        n215 = property class="Clust (strict)"(reference=w381, error in=w386, "Value"=w382) -> ()  [unwired: 2 out]
      }
      event "Single Jump C.Which Position to use for Experiment": Value Change {
        n216 = event-data() -> ()  [unwired: 1 in, 6 out]
        n217 = control-ref of="Single Jump C"() -> (w429:refnum<vi>)
        n218 = property class="Clust (strict)"(reference=w429) -> (error out=w433:errorcluster, "Value"=w428:T18)  [unwired: 1 in, 1 out]
        n219 = Unbundle By Name(w428) -> ("Which Position to use for Experiment"=w427:T28)
        n220 = case shown="\"Jumper Position o-C\"" w427 {
          tunnel: ["Experiment Safe Posistion" "Jumper Posistion A" "Jumper Posistion B" "Jumper Posistion B" "Jumper Posistion C" "wash" "Jumper Posistion C" "wash" "Jumper Posistion A" "Jumper Posistion A" "Jumper Safe Posistion" "Jumper Posistion B" "Jumper Posistion C"] -> w431
          tunnel: ["NA" "Jumper Posistion B" "Jumper Posistion A" "Jumper Posistion C" "Jumper Posistion B" "Jumper Posistion A" "wash" "Jumper Posistion C" "wash" "NA" "NA" "NA" "NA"] -> w432
          tunnel: w433 -> [w436 w440 w443 w446 w449 w451 w454 w457 w460 w463 w466 w469 w472]
          tunnel: [w436 w440 w443 w446 w449 w451 w454 w457 w460 w463 w466 w469 w472] -> w434
          frame "Experiment Safe Position" {
          }
          frame "Jumper Position A-B" {
          }
          frame "Jumper Position B-A" {
          }
          frame "Jumper Position B-C" {
          }
          frame "Jumper Position C-B" {
          }
          frame "Jumper Position o-A" {
          }
          frame "Jumper Position C-o" {
          }
          frame "Jumper Position o-C" {
          }
          frame "Jumper Position A-o" {
          }
          frame "Jumper Position A" {
          }
          frame "Jumper Safe Position" {
          }
          frame "Jumper Position B" {
          }
          frame "Jumper Position C" {
          }
        }
        n221 = Bundle By Name(cluster=w428, "Start Position (N)"=w431, "Jump Position (m)"=w432) -> (w430:T18)
        n222 = property class="Clust (strict)"(reference=w429, error in=w434, "Value"=w430) -> ()  [unwired: 2 out]
      }
      event "Single Jump D.Which Position to use for Experiment": Value Change {
        n223 = event-data() -> ()  [unwired: 1 in, 6 out]
        n224 = control-ref of="Single Jump D"() -> (w477:refnum<vi>)
        n225 = property class="Clust (strict)"(reference=w477) -> (error out=w481:errorcluster, "Value"=w476:T18)  [unwired: 1 in, 1 out]
        n226 = Unbundle By Name(w476) -> ("Which Position to use for Experiment"=w475:T28)
        n227 = case shown="\"Jumper Position o-C\"" w475 {
          tunnel: ["Experiment Safe Posistion" "Jumper Posistion A" "Jumper Posistion B" "Jumper Posistion B" "Jumper Posistion C" "wash" "Jumper Posistion C" "wash" "Jumper Posistion A" "Jumper Posistion A" "Jumper Safe Posistion" "Jumper Posistion B" "Jumper Posistion C"] -> w479
          tunnel: ["NA" "Jumper Posistion B" "Jumper Posistion A" "Jumper Posistion C" "Jumper Posistion B" "Jumper Posistion A" "wash" "Jumper Posistion C" "wash" "NA" "NA" "NA" "NA"] -> w480
          tunnel: w481 -> [w484 w488 w491 w494 w497 w499 w502 w505 w508 w511 w514 w517 w520]
          tunnel: [w484 w488 w491 w494 w497 w499 w502 w505 w508 w511 w514 w517 w520] -> w482
          frame "Experiment Safe Position" {
          }
          frame "Jumper Position A-B" {
          }
          frame "Jumper Position B-A" {
          }
          frame "Jumper Position B-C" {
          }
          frame "Jumper Position C-B" {
          }
          frame "Jumper Position o-A" {
          }
          frame "Jumper Position C-o" {
          }
          frame "Jumper Position o-C" {
          }
          frame "Jumper Position A-o" {
          }
          frame "Jumper Position A" {
          }
          frame "Jumper Safe Position" {
          }
          frame "Jumper Position B" {
          }
          frame "Jumper Position C" {
          }
        }
        n228 = Bundle By Name(cluster=w476, "Start Position (N)"=w479, "Jump Position (m)"=w480) -> (w478:T18)
        n229 = property class="Clust (strict)"(reference=w477, error in=w482, "Value"=w478) -> ()  [unwired: 2 out]
      }
      event "Single Jump E.Which Position to use for Experiment": Value Change {
        n230 = event-data() -> ()  [unwired: 1 in, 6 out]
        n231 = control-ref of="Single Jump E"() -> (w525:refnum<vi>)
        n232 = property class="Clust (strict)"(reference=w525) -> (error out=w529:errorcluster, "Value"=w524:T18)  [unwired: 1 in, 1 out]
        n233 = Unbundle By Name(w524) -> ("Which Position to use for Experiment"=w523:T28)
        n234 = case shown="\"Jumper Position o-C\"" w523 {
          tunnel: ["Experiment Safe Posistion" "Jumper Posistion A" "Jumper Posistion B" "Jumper Posistion B" "Jumper Posistion C" "wash" "Jumper Posistion C" "wash" "Jumper Posistion A" "Jumper Posistion A" "Jumper Safe Posistion" "Jumper Posistion B" "Jumper Posistion C"] -> w527
          tunnel: ["NA" "Jumper Posistion B" "Jumper Posistion A" "Jumper Posistion C" "Jumper Posistion B" "Jumper Posistion A" "wash" "Jumper Posistion C" "wash" "NA" "NA" "NA" "NA"] -> w528
          tunnel: w529 -> [w532 w536 w539 w542 w545 w547 w550 w553 w556 w559 w562 w565 w568]
          tunnel: [w532 w536 w539 w542 w545 w547 w550 w553 w556 w559 w562 w565 w568] -> w530
          frame "Experiment Safe Position" {
          }
          frame "Jumper Position A-B" {
          }
          frame "Jumper Position B-A" {
          }
          frame "Jumper Position B-C" {
          }
          frame "Jumper Position C-B" {
          }
          frame "Jumper Position o-A" {
          }
          frame "Jumper Position C-o" {
          }
          frame "Jumper Position o-C" {
          }
          frame "Jumper Position A-o" {
          }
          frame "Jumper Position A" {
          }
          frame "Jumper Safe Position" {
          }
          frame "Jumper Position B" {
          }
          frame "Jumper Position C" {
          }
        }
        n235 = Bundle By Name(cluster=w524, "Start Position (N)"=w527, "Jump Position (m)"=w528) -> (w526:T18)
        n236 = property class="Clust (strict)"(reference=w525, error in=w530, "Value"=w526) -> ()  [unwired: 2 out]
      }
      event "Single Jump F.Which Position to use for Experiment": Value Change {
        n237 = event-data() -> ()  [unwired: 1 in, 6 out]
        n238 = control-ref of="Single Jump F"() -> (w573:refnum<vi>)
        n239 = property class="Clust (strict)"(reference=w573) -> (error out=w577:errorcluster, "Value"=w572:T18)  [unwired: 1 in, 1 out]
        n240 = Unbundle By Name(w572) -> ("Which Position to use for Experiment"=w571:T28)
        n241 = case shown="\"Jumper Position o-C\"" w571 {
          tunnel: ["Experiment Safe Posistion" "Jumper Posistion A" "Jumper Posistion B" "Jumper Posistion B" "Jumper Posistion C" "wash" "Jumper Posistion C" "wash" "Jumper Posistion A" "Jumper Posistion A" "Jumper Safe Posistion" "Jumper Posistion B" "Jumper Posistion C"] -> w575
          tunnel: ["NA" "Jumper Posistion B" "Jumper Posistion A" "Jumper Posistion C" "Jumper Posistion B" "Jumper Posistion A" "wash" "Jumper Posistion C" "wash" "NA" "NA" "NA" "NA"] -> w576
          tunnel: w577 -> [w580 w584 w587 w590 w593 w595 w598 w601 w604 w607 w610 w613 w616]
          tunnel: [w580 w584 w587 w590 w593 w595 w598 w601 w604 w607 w610 w613 w616] -> w578
          frame "Experiment Safe Position" {
          }
          frame "Jumper Position A-B" {
          }
          frame "Jumper Position B-A" {
          }
          frame "Jumper Position B-C" {
          }
          frame "Jumper Position C-B" {
          }
          frame "Jumper Position o-A" {
          }
          frame "Jumper Position C-o" {
          }
          frame "Jumper Position o-C" {
          }
          frame "Jumper Position A-o" {
          }
          frame "Jumper Position A" {
          }
          frame "Jumper Safe Position" {
          }
          frame "Jumper Position B" {
          }
          frame "Jumper Position C" {
          }
        }
        n242 = Bundle By Name(cluster=w572, "Start Position (N)"=w575, "Jump Position (m)"=w576) -> (w574:T18)
        n243 = property class="Clust (strict)"(reference=w573, error in=w578, "Value"=w574) -> ()  [unwired: 2 out]
      }
      event "update plots": Value Change {
        n244 = event-data() -> ("NewVal"=w620:bool)  [unwired: 1 in, 5 out]
        n245 = case shown="True" w620 {
          tunnel: w619 -> [_ w623]
          tunnel: [FALSE w622] -> w618
          frame False {
          }
          frame True {
            n246 = stacked-sequence {
              tunnel: w623 -> [w630 w631 _ _ _ _ _]
              tunnel: [_ _ _ _ _ _ w654] -> w622
              frame #0 {
                # "repMemTest Iprot"
                n247 = local read "repMemTest Iprot"() -> (w628:T12)
                n248 = Unbundle By Name(w628) -> ("Iclamp in"=w627:T11, "# iter"=w626:i32, "# reps IC"=w625:i32)
                n249 = call "clamp_protocol.vi"("which clamp"=enum16{"VClamp", "IClamp"}."IClamp", "# reps"=w625, "# Iterations"=w626, "clamp in"=w627, "sampling rate (Hz)"=w630) -> ("View profile (wvfrms)"=→"repMemTest iprot cmd":waveform(dbl)[])  [unwired: 2 out]
              }
              frame #1 {
                # "repMemTest Vprot"
                n250 = local read "repMemTest Vprot"() -> (w635:T13)
                n251 = Unbundle By Name(w635) -> ("Vclamp in"=w636:T11, "# iter"=w633:i32, "# reps VC"=w632:i32)
                n252 = call "clamp_protocol.vi"("which clamp"=enum16{"VClamp", "IClamp"}."VClamp", "# reps"=w632, "# Iterations"=w633, "clamp in"=w636, "sampling rate (Hz)"=w631) -> ("View profile (wvfrms)"=→"repMemTest vprot cmd":waveform(dbl)[])  [unwired: 2 out]
              }
              frame #2 {
                # "repMemTest Imem"
                n253 = local read "repMemTest Iclamp memtest"() -> (w638:T14)
                n254 = call "ext_cmd_sensitivity.vi"("which clamp"=enum16{"VClamp", "IClamp"}."IClamp") -> ("division factor"=w641:dbl)  [unwired: 10 in]
                n255 = call "generate_memtest_pulse.vi"("external cmd sensitivity"=w641, "memtest"=w638) -> ("view memtest"=→"repMemTest imemtest view":waveform(dbl))  [unwired: 8 in, 1 out]
              }
              frame #3 {
                # "repMemTest Vmem"
                n256 = local read "repMemTest Vclamp memtest"() -> (w642:T14)
                n257 = call "ext_cmd_sensitivity.vi"("which clamp"=enum16{"VClamp", "IClamp"}."VClamp") -> ("division factor"=w645:dbl)  [unwired: 10 in]
                n258 = call "generate_memtest_pulse.vi"("external cmd sensitivity"=w645, "memtest"=w642) -> ("view memtest"=→"repMemTest vmemtest view":waveform(dbl))  [unwired: 8 in, 1 out]
              }
              frame #4 {
                # "Holding Imem"
                n259 = local read "holding Iclamp memtest"() -> (w646:T14)
                n260 = call "ext_cmd_sensitivity.vi"("which clamp"=enum16{"VClamp", "IClamp"}."IClamp") -> ("division factor"=w649:dbl)  [unwired: 10 in]
                n261 = call "generate_memtest_pulse.vi"("external cmd sensitivity"=w649, "memtest"=w646) -> ("view memtest"=→"holding imemtest cmd":waveform(dbl))  [unwired: 8 in, 1 out]
              }
              frame #5 {
                # "Holding Vmem"
                n262 = local read "holding Vclamp memtest"() -> (w650:T14)
                n263 = call "ext_cmd_sensitivity.vi"("which clamp"=enum16{"VClamp", "IClamp"}."VClamp") -> ("division factor"=w653:dbl)  [unwired: 10 in]
                n264 = call "generate_memtest_pulse.vi"("external cmd sensitivity"=w653, "memtest"=w650) -> ("view memtest"=→"holding vmemtest cmd":waveform(dbl))  [unwired: 8 in, 1 out]
              }
              frame #6 {
                n265 = local read "auto run?"() -> (w655:bool)
                n266 = case shown="True" w655 {
                  tunnel: [FALSE TRUE] -> w654
                  frame False {
                  }
                  frame True {
                    n267 = local write "auto WC run trigger"(TRUE ("auto WC run trigger")) -> ()
                    n268 = property on="update plots" class="Bool (strict)"("Value"=FALSE ("Value (Signaling)")) -> ()  [unwired: 2 in, 2 out]
                  }
                }
              }
            }
          }
        }
      }
      event "run": Value Change {
        n269 = event-data() -> ("NewVal"=w661:bool)  [unwired: 1 in, 5 out]
        n270 = case shown="True" w661 {
          selector: w661 -> [_ w662]
          frame False {
          }
          frame True {
            n271 = property on="auto WC run trigger" class="Bool (strict)"("Value"=w662) -> ()  [unwired: 2 in, 2 out]
          }
        }
      }
      event "save", "save as...": Value Change {
        n272 = event-data() -> ("NewVal"=w664:bool)  [unwired: 1 in, 5 out]
        n273 = case shown="True" w664 {
          tunnel: "save as..." -> [_ w672]
          tunnel: w666 -> [_ w671]
          tunnel: w665 -> [_ w670]
          frame False {
          }
          frame True {
            n274 = case shown="True" w672 {
              tunnel: w671 -> [w678 _]
              tunnel: [w678 w680] -> w669
              tunnel: [FALSE ("cancelled") w679] -> w668
              frame False {
              }
              frame True {
                n275 = call "select config"("prompt"="Save as...") -> ("selected path"=w680:path, "cancelled"=w679:bool)  [unwired: 11 in, 2 out]
                n276 = local write "config file"(w680) -> ()
              }
            }
            n277 = case shown="False" w668 {
              tunnel: w670 -> [w674 _]
              tunnel: w669 -> [w675 _]
              frame False {
                n278 = call "condition_control_array.vi"("control array in"=w674) -> ("control array out"=w673:refnum<vi>[])  [unwired: 9 in, 1 out]
                n279 = call "Read and Write Controls to Automatic Config File.vi"("Action"=RWC_Actions."Write", "Control References"=w673, "filepath"=w675) -> ()  [unwired: 8 in, 1 out]
              }
              frame True {
              }
            }
          }
        }
      }
      event "load": Value Change {
        n280 = event-data() -> ("NewVal"=w684:bool)  [unwired: 1 in, 5 out]
        n281 = case shown="True" w684 {
          tunnel: w683 -> [_ w687]
          frame False {
          }
          frame True {
            n282 = call "load config"() -> ("selected path"=w686:path, "cancelled"=w685:bool)  [unwired: 12 in, 2 out]
            n283 = case shown="False" w685 {
              tunnel: w687 -> [w690 _]
              tunnel: w686 -> [w688 _]
              frame False {
                n284 = call "Read and Write Controls to Automatic Config File.vi"("Action"=RWC_Actions."Read", "Control References"=w690, "filepath"=w688) -> ()  [unwired: 8 in, 1 out]
                n285 = local write "config file"(w688) -> ()
              }
              frame True {
              }
            }
          }
        }
      }
    }
  }
  n286 = control-ref of="PhaseA Experiment Option"() -> (w77:refnum<vi>)
  n287 = control-ref of="Single Manip Jump A"() -> (w61:refnum<vi>)
  n288 = control-ref of="Paired Pulse A"() -> (w76:refnum<vi>)
  n289 = control-ref of="Jump Train A"() -> (w75:refnum<vi>)
  n290 = control-ref of="Voltage Ramp A"() -> (w74:refnum<vi>)
  n291 = control-ref of="Voltage Step A"() -> (w73:refnum<vi>)
  n292 = control-ref of="Solution Change A"() -> (w72:refnum<vi>)
  n293 = control-ref of="Single Jump A"() -> (w71:refnum<vi>)
  n294 = Bundle(cluster="PhaseX Cluster", "Phase Experiment Option"=w77, "Paired Pulse"=w76, "Jump Train"=w75, "Voltage Ramp"=w74, "Voltage Step"=w73, "Solution Change"=w72, "Single Jump"=w71, "Single Manip Jump"=w61) -> (w60:T1)
  n295 = control-ref of="PhaseB Experiment Option"() -> (w70:refnum<vi>)
  n296 = control-ref of="Paired Pulse B"() -> (w64:refnum<vi>)
  n297 = control-ref of="Jump Train B"() -> (w65:refnum<vi>)
  n298 = control-ref of="Voltage Ramp B"() -> (w66:refnum<vi>)
  n299 = control-ref of="Voltage Step B"() -> (w67:refnum<vi>)
  n300 = control-ref of="Solution Change B"() -> (w68:refnum<vi>)
  n301 = control-ref of="Single Jump B"() -> (w69:refnum<vi>)
  n302 = control-ref of="Single Manip Jump B"() -> (w62:refnum<vi>)
  n303 = Bundle(cluster="PhaseX Cluster", "Phase Experiment Option"=w70, "Paired Pulse"=w64, "Jump Train"=w65, "Voltage Ramp"=w66, "Voltage Step"=w67, "Solution Change"=w68, "Single Jump"=w69, "Single Manip Jump"=w62) -> (w59:T1)
  n304 = control-ref of="PhaseC Experiment Option"() -> (w56:refnum<vi>)
  n305 = control-ref of="Paired Pulse C"() -> (w55:refnum<vi>)
  n306 = control-ref of="Jump Train C"() -> (w54:refnum<vi>)
  n307 = control-ref of="Voltage Ramp C"() -> (w53:refnum<vi>)
  n308 = control-ref of="Voltage Step C"() -> (w52:refnum<vi>)
  n309 = control-ref of="Solution Change C"() -> (w51:refnum<vi>)
  n310 = control-ref of="Single Jump C"() -> (w50:refnum<vi>)
  n311 = control-ref of="Single Manip Jump C"() -> (w49:refnum<vi>)
  n312 = Bundle(cluster="PhaseX Cluster", "Phase Experiment Option"=w56, "Paired Pulse"=w55, "Jump Train"=w54, "Voltage Ramp"=w53, "Voltage Step"=w52, "Solution Change"=w51, "Single Jump"=w50, "Single Manip Jump"=w49) -> (w48:T1)
  n313 = while {
    stop <- w697 stop-if-true
    n314 = control-ref of="common cluster"() -> (w699:refnum<vi>)
    n315 = property class="Clust (strict)"(reference=w699) -> ("Value"=w695:T6)  [unwired: 1 in, 2 out]
    n316 = Unbundle By Name(w695) -> ("positioning+hunting common.transforms"=w704:refnum<vi>)
    n317 = local read "Running"() -> (w701:bool)
    n318 = Wait (ms)(milliseconds to wait=u32 100) -> ()  [unwired: 1 out]
    n319 = property class="Clust (strict)"(reference=w704) -> (error out=w710:errorcluster, "Value"=w703:T29)  [unwired: 1 in, 1 out]
    n320 = local read "Experiment Done"() -> (w696:bool)
    n321 = Unbundle By Name(w703) -> ("manip 1"=w702:refnum<vi>)
    n322 = property class="Clust (strict)"(reference=w702, error in=w710) -> (error out=w711:errorcluster, "Value"=w708:T30)  [unwired: 1 out]
    n323 = Unbundle By Name(w708) -> ("actuator"=w709:T31)
    n324 = call "get_XYZ.vi"("Actuator cluster in"=w709, "error in"=w711) -> ("X pos (steps)"=w705:i32, "Y pos (steps)"=w706:i32, "Z pos (steps)"=w707:i32)  [unwired: 9 in, 2 out]
    n325 = Not(x=w701) -> (.not. x?=w700:bool)
    n326 = Or(x=w696, y=w700) -> (x .or. y?=w697:bool)
    n327 = Build Array(w705, w706, w707) -> (w692:i32[])
    n328 = Divide(x=w692, y=10) -> (x/y=w694:dbl[])
    n329 = To Long Integer(number=w694) -> (32bit integer=w691:i32[])
    "Current Manipulator Position [uM]" <- w691
    n330 = stacked-sequence {
      tunnel: w695 -> [_ w730 w749 w768 w787 w806 w825 w844 w863 w882 w901 w920 w939 w958]
      tunnel: w691 -> [_ w713 w732 w754 w770 w789 w808 w827 w846 w865 w884 w903 w922 w941]
      frame #0 {
        n331 = local write "Current Position"("" ("Current Position")) -> ()
      }
      frame #1 {
        n332 = Unbundle By Name(w730) -> ("JumperPositions.jumperSafePos"=w729:refnum<vi>)
        n333 = property class="Arr (strict)"(reference=w729) -> ("Value"=w715:dbl[], "Caption.Text"=w718:string)  [unwired: 1 in, 2 out]
        n334 = Index Array(array=w713) -> (element #1=w727:i32, element #2=w725:i32, element #3=w724:i32)  [unwired: 3 in]
        n335 = Divide(x=w715, y=10) -> (x/y=w716:dbl[])
        n336 = To Long Integer(number=w716) -> (32bit integer=w714:i32[])
        n337 = Index Array(array=w714) -> (element #1=w728:i32, element #2=w726:i32, element #3=w723:i32)  [unwired: 3 in]
        n338 = Equal?(x=w728, y=w727) -> (x = y?=w722:bool)
        n339 = Equal?(x=w726, y=w725) -> (x = y?=w721:bool)
        n340 = Equal?(x=w723, y=w724) -> (x = y?=w720:bool)
        n341 = Compound Arithmetic op=AND(w722, w721, w720) -> (w719:bool)
        n342 = case shown="True" w719 {
          tunnel: w718 -> [_ w731]
          frame False {
          }
          frame True {
            n343 = local write "Current Position"(w731) -> ()
          }
        }
      }
      frame #2 {
        n344 = Unbundle By Name(w749) -> ("JumperPositions.ExpSafePos"=w748:refnum<vi>)
        n345 = property class="Arr (strict)"(reference=w748) -> ("Value"=w734:dbl[], "Caption.Text"=w737:string)  [unwired: 1 in, 2 out]
        n346 = Index Array(array=w732) -> (element #1=w746:i32, element #2=w744:i32, element #3=w743:i32)  [unwired: 3 in]
        n347 = Divide(x=w734, y=10) -> (x/y=w735:dbl[])
        n348 = To Long Integer(number=w735) -> (32bit integer=w733:i32[])
        n349 = Index Array(array=w733) -> (element #1=w747:i32, element #2=w745:i32, element #3=w742:i32)  [unwired: 3 in]
        n350 = Equal?(x=w747, y=w746) -> (x = y?=w741:bool)
        n351 = Equal?(x=w745, y=w744) -> (x = y?=w740:bool)
        n352 = Equal?(x=w742, y=w743) -> (x = y?=w739:bool)
        n353 = Compound Arithmetic op=AND(w741, w740, w739) -> (w738:bool)
        n354 = case shown="True" w738 {
          tunnel: w737 -> [_ w750]
          frame False {
          }
          frame True {
            n355 = local write "Current Position"(w750) -> ()
          }
        }
      }
      frame #3 {
        n356 = Unbundle By Name(w768) -> ("JumperPositions.JumperPos A"=w767:refnum<vi>)
        n357 = property class="Arr (strict)"(reference=w767) -> ("Value"=w751:dbl[], "Caption.Text"=w756:string)  [unwired: 1 in, 2 out]
        n358 = Index Array(array=w754) -> (element #1=w765:i32, element #2=w763:i32, element #3=w762:i32)  [unwired: 3 in]
        n359 = Divide(x=w751, y=10) -> (x/y=w752:dbl[])
        n360 = To Long Integer(number=w752) -> (32bit integer=w753:i32[])
        n361 = Index Array(array=w753) -> (element #1=w766:i32, element #2=w764:i32, element #3=w761:i32)  [unwired: 3 in]
        n362 = Equal?(x=w766, y=w765) -> (x = y?=w760:bool)
        n363 = Equal?(x=w764, y=w763) -> (x = y?=w759:bool)
        n364 = Equal?(x=w761, y=w762) -> (x = y?=w758:bool)
        n365 = Compound Arithmetic op=AND(w760, w759, w758) -> (w757:bool)
        n366 = case shown="True" w757 {
          tunnel: w756 -> [_ w769]
          frame False {
          }
          frame True {
            n367 = local write "Current Position"(w769) -> ()
          }
        }
      }
      frame #4 {
        n368 = Unbundle By Name(w787) -> ("JumperPositions.JumperPos B"=w786:refnum<vi>)
        n369 = property class="Arr (strict)"(reference=w786) -> ("Value"=w772:dbl[], "Caption.Text"=w775:string)  [unwired: 1 in, 2 out]
        n370 = Index Array(array=w770) -> (element #1=w784:i32, element #2=w782:i32, element #3=w781:i32)  [unwired: 3 in]
        n371 = Divide(x=w772, y=10) -> (x/y=w773:dbl[])
        n372 = To Long Integer(number=w773) -> (32bit integer=w771:i32[])
        n373 = Index Array(array=w771) -> (element #1=w785:i32, element #2=w783:i32, element #3=w780:i32)  [unwired: 3 in]
        n374 = Equal?(x=w785, y=w784) -> (x = y?=w779:bool)
        n375 = Equal?(x=w783, y=w782) -> (x = y?=w778:bool)
        n376 = Equal?(x=w780, y=w781) -> (x = y?=w777:bool)
        n377 = Compound Arithmetic op=AND(w779, w778, w777) -> (w776:bool)
        n378 = case shown="True" w776 {
          tunnel: w775 -> [_ w788]
          frame False {
          }
          frame True {
            n379 = local write "Current Position"(w788) -> ()
          }
        }
      }
      frame #5 {
        n380 = Unbundle By Name(w806) -> ("JumperPositions.JumperPos C"=w805:refnum<vi>)
        n381 = property class="Arr (strict)"(reference=w805) -> ("Value"=w791:dbl[], "Caption.Text"=w794:string)  [unwired: 1 in, 2 out]
        n382 = Index Array(array=w789) -> (element #1=w803:i32, element #2=w801:i32, element #3=w800:i32)  [unwired: 3 in]
        n383 = Divide(x=w791, y=10) -> (x/y=w792:dbl[])
        n384 = To Long Integer(number=w792) -> (32bit integer=w790:i32[])
        n385 = Index Array(array=w790) -> (element #1=w804:i32, element #2=w802:i32, element #3=w799:i32)  [unwired: 3 in]
        n386 = Equal?(x=w804, y=w803) -> (x = y?=w798:bool)
        n387 = Equal?(x=w802, y=w801) -> (x = y?=w797:bool)
        n388 = Equal?(x=w799, y=w800) -> (x = y?=w796:bool)
        n389 = Compound Arithmetic op=AND(w798, w797, w796) -> (w795:bool)
        n390 = case shown="True" w795 {
          tunnel: w794 -> [_ w807]
          frame False {
          }
          frame True {
            n391 = local write "Current Position"(w807) -> ()
          }
        }
      }
      frame #6 {
        n392 = Unbundle By Name(w825) -> ("JumperPositions.JumperPos o-A"=w824:refnum<vi>)
        n393 = property class="Arr (strict)"(reference=w824) -> ("Value"=w810:dbl[], "Caption.Text"=w813:string)  [unwired: 1 in, 2 out]
        n394 = Index Array(array=w808) -> (element #1=w822:i32, element #2=w820:i32, element #3=w819:i32)  [unwired: 3 in]
        n395 = Divide(x=w810, y=10) -> (x/y=w811:dbl[])
        n396 = To Long Integer(number=w811) -> (32bit integer=w809:i32[])
        n397 = Index Array(array=w809) -> (element #1=w823:i32, element #2=w821:i32, element #3=w818:i32)  [unwired: 3 in]
        n398 = Equal?(x=w823, y=w822) -> (x = y?=w817:bool)
        n399 = Equal?(x=w821, y=w820) -> (x = y?=w816:bool)
        n400 = Equal?(x=w818, y=w819) -> (x = y?=w815:bool)
        n401 = Compound Arithmetic op=AND(w817, w816, w815) -> (w814:bool)
        n402 = case shown="True" w814 {
          tunnel: w813 -> [_ w826]
          frame False {
          }
          frame True {
            n403 = local write "Current Position"(w826) -> ()
          }
        }
      }
      frame #7 {
        n404 = Unbundle By Name(w844) -> ("JumperPositions.JumperPos A-o"=w843:refnum<vi>)
        n405 = property class="Arr (strict)"(reference=w843) -> ("Value"=w829:dbl[], "Caption.Text"=w832:string)  [unwired: 1 in, 2 out]
        n406 = Index Array(array=w827) -> (element #1=w841:i32, element #2=w839:i32, element #3=w838:i32)  [unwired: 3 in]
        n407 = Divide(x=w829, y=10) -> (x/y=w830:dbl[])
        n408 = To Long Integer(number=w830) -> (32bit integer=w828:i32[])
        n409 = Index Array(array=w828) -> (element #1=w842:i32, element #2=w840:i32, element #3=w837:i32)  [unwired: 3 in]
        n410 = Equal?(x=w842, y=w841) -> (x = y?=w836:bool)
        n411 = Equal?(x=w840, y=w839) -> (x = y?=w835:bool)
        n412 = Equal?(x=w837, y=w838) -> (x = y?=w834:bool)
        n413 = Compound Arithmetic op=AND(w836, w835, w834) -> (w833:bool)
        n414 = case shown="True" w833 {
          tunnel: w832 -> [_ w845]
          frame False {
          }
          frame True {
            n415 = local write "Current Position"(w845) -> ()
          }
        }
      }
      frame #8 {
        n416 = Unbundle By Name(w863) -> ("JumperPositions.JumperPos A-B"=w862:refnum<vi>)
        n417 = property class="Arr (strict)"(reference=w862) -> ("Value"=w848:dbl[], "Caption.Text"=w851:string)  [unwired: 1 in, 2 out]
        n418 = Index Array(array=w846) -> (element #1=w860:i32, element #2=w858:i32, element #3=w857:i32)  [unwired: 3 in]
        n419 = Divide(x=w848, y=10) -> (x/y=w849:dbl[])
        n420 = To Long Integer(number=w849) -> (32bit integer=w847:i32[])
        n421 = Index Array(array=w847) -> (element #1=w861:i32, element #2=w859:i32, element #3=w856:i32)  [unwired: 3 in]
        n422 = Equal?(x=w861, y=w860) -> (x = y?=w855:bool)
        n423 = Equal?(x=w859, y=w858) -> (x = y?=w854:bool)
        n424 = Equal?(x=w856, y=w857) -> (x = y?=w853:bool)
        n425 = Compound Arithmetic op=AND(w855, w854, w853) -> (w852:bool)
        n426 = case shown="True" w852 {
          tunnel: w851 -> [_ w864]
          frame False {
          }
          frame True {
            n427 = local write "Current Position"(w864) -> ()
          }
        }
      }
      frame #9 {
        n428 = Unbundle By Name(w882) -> ("JumperPositions.JumperPos B-A"=w881:refnum<vi>)
        n429 = property class="Arr (strict)"(reference=w881) -> ("Value"=w867:dbl[], "Caption.Text"=w870:string)  [unwired: 1 in, 2 out]
        n430 = Index Array(array=w865) -> (element #1=w879:i32, element #2=w877:i32, element #3=w876:i32)  [unwired: 3 in]
        n431 = Divide(x=w867, y=10) -> (x/y=w868:dbl[])
        n432 = To Long Integer(number=w868) -> (32bit integer=w866:i32[])
        n433 = Index Array(array=w866) -> (element #1=w880:i32, element #2=w878:i32, element #3=w875:i32)  [unwired: 3 in]
        n434 = Equal?(x=w880, y=w879) -> (x = y?=w874:bool)
        n435 = Equal?(x=w878, y=w877) -> (x = y?=w873:bool)
        n436 = Equal?(x=w875, y=w876) -> (x = y?=w872:bool)
        n437 = Compound Arithmetic op=AND(w874, w873, w872) -> (w871:bool)
        n438 = case shown="True" w871 {
          tunnel: w870 -> [_ w883]
          frame False {
          }
          frame True {
            n439 = local write "Current Position"(w883) -> ()
          }
        }
      }
      frame #10 {
        n440 = Unbundle By Name(w901) -> ("JumperPositions.JumperPos B-C"=w900:refnum<vi>)
        n441 = property class="Arr (strict)"(reference=w900) -> ("Value"=w886:dbl[], "Caption.Text"=w889:string)  [unwired: 1 in, 2 out]
        n442 = Index Array(array=w884) -> (element #1=w898:i32, element #2=w896:i32, element #3=w895:i32)  [unwired: 3 in]
        n443 = Divide(x=w886, y=10) -> (x/y=w887:dbl[])
        n444 = To Long Integer(number=w887) -> (32bit integer=w885:i32[])
        n445 = Index Array(array=w885) -> (element #1=w899:i32, element #2=w897:i32, element #3=w894:i32)  [unwired: 3 in]
        n446 = Equal?(x=w899, y=w898) -> (x = y?=w893:bool)
        n447 = Equal?(x=w897, y=w896) -> (x = y?=w892:bool)
        n448 = Equal?(x=w894, y=w895) -> (x = y?=w891:bool)
        n449 = Compound Arithmetic op=AND(w893, w892, w891) -> (w890:bool)
        n450 = case shown="True" w890 {
          tunnel: w889 -> [_ w902]
          frame False {
          }
          frame True {
            n451 = local write "Current Position"(w902) -> ()
          }
        }
      }
      frame #11 {
        n452 = Unbundle By Name(w920) -> ("JumperPositions.JumperPos C-B"=w919:refnum<vi>)
        n453 = property class="Arr (strict)"(reference=w919) -> ("Value"=w905:dbl[], "Caption.Text"=w908:string)  [unwired: 1 in, 2 out]
        n454 = Index Array(array=w903) -> (element #1=w917:i32, element #2=w915:i32, element #3=w914:i32)  [unwired: 3 in]
        n455 = Divide(x=w905, y=10) -> (x/y=w906:dbl[])
        n456 = To Long Integer(number=w906) -> (32bit integer=w904:i32[])
        n457 = Index Array(array=w904) -> (element #1=w918:i32, element #2=w916:i32, element #3=w913:i32)  [unwired: 3 in]
        n458 = Equal?(x=w918, y=w917) -> (x = y?=w912:bool)
        n459 = Equal?(x=w916, y=w915) -> (x = y?=w911:bool)
        n460 = Equal?(x=w913, y=w914) -> (x = y?=w910:bool)
        n461 = Compound Arithmetic op=AND(w912, w911, w910) -> (w909:bool)
        n462 = case shown="True" w909 {
          tunnel: w908 -> [_ w921]
          frame False {
          }
          frame True {
            n463 = local write "Current Position"(w921) -> ()
          }
        }
      }
      frame #12 {
        n464 = Unbundle By Name(w939) -> ("JumperPositions.JumperPos C-o"=w938:refnum<vi>)
        n465 = property class="Arr (strict)"(reference=w938) -> ("Value"=w924:dbl[], "Caption.Text"=w927:string)  [unwired: 1 in, 2 out]
        n466 = Index Array(array=w922) -> (element #1=w936:i32, element #2=w934:i32, element #3=w933:i32)  [unwired: 3 in]
        n467 = Divide(x=w924, y=10) -> (x/y=w925:dbl[])
        n468 = To Long Integer(number=w925) -> (32bit integer=w923:i32[])
        n469 = Index Array(array=w923) -> (element #1=w937:i32, element #2=w935:i32, element #3=w932:i32)  [unwired: 3 in]
        n470 = Equal?(x=w937, y=w936) -> (x = y?=w931:bool)
        n471 = Equal?(x=w935, y=w934) -> (x = y?=w930:bool)
        n472 = Equal?(x=w932, y=w933) -> (x = y?=w929:bool)
        n473 = Compound Arithmetic op=AND(w931, w930, w929) -> (w928:bool)
        n474 = case shown="True" w928 {
          tunnel: w927 -> [_ w940]
          frame False {
          }
          frame True {
            n475 = local write "Current Position"(w940) -> ()
          }
        }
      }
      frame #13 {
        n476 = Unbundle By Name(w958) -> ("JumperPositions.JumperPos o-C"=w957:refnum<vi>)
        n477 = property class="Arr (strict)"(reference=w957) -> ("Value"=w943:dbl[], "Caption.Text"=w946:string)  [unwired: 1 in, 2 out]
        n478 = Index Array(array=w941) -> (element #1=w955:i32, element #2=w953:i32, element #3=w952:i32)  [unwired: 3 in]
        n479 = Divide(x=w943, y=10) -> (x/y=w944:dbl[])
        n480 = To Long Integer(number=w944) -> (32bit integer=w942:i32[])
        n481 = Index Array(array=w942) -> (element #1=w956:i32, element #2=w954:i32, element #3=w951:i32)  [unwired: 3 in]
        n482 = Equal?(x=w956, y=w955) -> (x = y?=w950:bool)
        n483 = Equal?(x=w954, y=w953) -> (x = y?=w949:bool)
        n484 = Equal?(x=w951, y=w952) -> (x = y?=w948:bool)
        n485 = Compound Arithmetic op=AND(w950, w949, w948) -> (w947:bool)
        n486 = case shown="True" w947 {
          tunnel: w946 -> [_ w959]
          frame False {
          }
          frame True {
            n487 = local write "Current Position"(w959) -> ()
          }
        }
      }
    }
  }
  n488 = control-ref of="PhaseD Experiment Option"() -> (w32:refnum<vi>)
  n489 = control-ref of="Paired Pulse D"() -> (w31:refnum<vi>)
  n490 = control-ref of="Jump Train D"() -> (w30:refnum<vi>)
  n491 = control-ref of="Voltage Ramp D"() -> (w29:refnum<vi>)
  n492 = control-ref of="Voltage Step D"() -> (w28:refnum<vi>)
  n493 = control-ref of="Solution Change D"() -> (w27:refnum<vi>)
  n494 = control-ref of="Single Jump D"() -> (w26:refnum<vi>)
  n495 = control-ref of="Single Manip Jump D"() -> (w25:refnum<vi>)
  n496 = Bundle(cluster="PhaseX Cluster", "Phase Experiment Option"=w32, "Paired Pulse"=w31, "Jump Train"=w30, "Voltage Ramp"=w29, "Voltage Step"=w28, "Solution Change"=w27, "Single Jump"=w26, "Single Manip Jump"=w25) -> (w7:T1)
  n497 = control-ref of="PhaseE Experiment Option"() -> (w23:refnum<vi>)
  n498 = control-ref of="Paired Pulse E"() -> (w22:refnum<vi>)
  n499 = control-ref of="Jump Train E"() -> (w21:refnum<vi>)
  n500 = control-ref of="Voltage Ramp E"() -> (w20:refnum<vi>)
  n501 = control-ref of="Voltage Step E"() -> (w19:refnum<vi>)
  n502 = control-ref of="Solution Change E"() -> (w18:refnum<vi>)
  n503 = control-ref of="Single Jump E"() -> (w17:refnum<vi>)
  n504 = control-ref of="Single Manip Jump E"() -> (w16:refnum<vi>)
  n505 = Bundle(cluster="PhaseX Cluster", "Phase Experiment Option"=w23, "Paired Pulse"=w22, "Jump Train"=w21, "Voltage Ramp"=w20, "Voltage Step"=w19, "Solution Change"=w18, "Single Jump"=w17, "Single Manip Jump"=w16) -> (w6:T1)
  n506 = control-ref of="PhaseF Experiment Option"() -> (w15:refnum<vi>)
  n507 = control-ref of="Paired Pulse F"() -> (w14:refnum<vi>)
  n508 = control-ref of="Jump Train F"() -> (w13:refnum<vi>)
  n509 = control-ref of="Voltage Ramp F"() -> (w12:refnum<vi>)
  n510 = control-ref of="Voltage Step F"() -> (w11:refnum<vi>)
  n511 = control-ref of="Solution Change F"() -> (w10:refnum<vi>)
  n512 = control-ref of="Single Jump F"() -> (w9:refnum<vi>)
  n513 = control-ref of="Single Manip Jump F"() -> (w8:refnum<vi>)
  n514 = Bundle(cluster="PhaseX Cluster", "Phase Experiment Option"=w15, "Paired Pulse"=w14, "Jump Train"=w13, "Voltage Ramp"=w12, "Voltage Step"=w11, "Solution Change"=w10, "Single Jump"=w9, "Single Manip Jump"=w8) -> (w5:T1)
  n515 = Bundle(cluster="ExperimentOptionsCluster", "How Many Experimental Phases?"=refnum<vi> refnum, "PhaseA Cluster"=w60, "PhaseB Cluster"=w59, "PhaseC Cluster"=w48, "PhaseD Cluster"=w7, "PhaseE Cluster"=w6, "PhaseF Cluster"=w5) -> (w47:T2)
  n516 = while {
    tunnel: w107 -> [w961]
    tunnel: w106 -> [w960]
    tunnel: w100 -> [w975]
    tunnel: w102 -> [w974]
    tunnel: [w965] -> w44
    tunnel: w39 -> [w972]
    tunnel: "common cluster" -> [w967]
    tunnel: "individual controls in" -> [w971]
    tunnel: "images" -> [w970]
    tunnel: "which manipulator" -> [w969]
    tunnel: w47 -> [w968]
    tunnel: w42 -> [w962]
    stop <- w966 stop-if-true
    # "Experiment"
    # "images"
    # "individual"
    # "Common"
    n517 = case shown="True" "auto WC run trigger" {
      tunnel: w975 -> [_ w1020]
      tunnel: w974 -> [_ w1012]
      tunnel: [w978 w993] -> w965
      tunnel: w972 -> [w978 w997]
      tunnel: w967 -> [_ w1003]
      tunnel: w971 -> [_ w1002]
      tunnel: w970 -> [_ _]
      tunnel: w969 -> [_ w1001]
      tunnel: w968 -> [_ w1004]
      tunnel: [FALSE ("Experiment Done") w992] -> w964
      tunnel: w962 -> [_ w984]
      tunnel: w961 -> [_ w982]
      tunnel: w960 -> [_ w981]
      frame False {
        # "if not running auto WC, wait 200 ms"
        n518 = Wait (ms)(milliseconds to wait=u32 200) -> ()  [unwired: 1 out]
      }
      frame True {
        # "write the whole config to the experiment day folder"
        n519 = call "set_status_string.vi"("error in"=w997, "new line?"=TRUE, "status string in"="~~~AUTO RUN ON~~~", "controls array"=w1020) -> ("error out"=w1010:errorcluster, "controls array out"=w1007:refnum<vi>[])  [unwired: 6 in]
        n520 = call "run_repeatingMembraneTest_pharmabot.vi"("ExpPhase"="preLift", "error in"=w1010, "data in"=w1012, "misc common.stop memtest"=w984, "controls array in"=w1007) -> ("error out"=w1009:errorcluster, "data out"=w1011:T9, "control array out"=w1000:refnum<vi>[])  [unwired: 2 in, 2 out]
        n521 = call "run_repeatingMembraneTest_pharmabot.vi"("ExpPhase"="postLift", "error in"=w1009, "data in"=w1011, "misc common.stop memtest"=w984, "controls array in"=w1000) -> ("error out"=w1005:errorcluster, "data out"=w1006:T9, "Cell Good?"=w980:bool, "control array out"=w999:refnum<vi>[])  [unwired: 2 in, 1 out]
        n522 = case shown="True" w980 {
          tunnel: w1006 -> [w1027 w1047]
          tunnel: w1005 -> [w1025 w1044]
          tunnel: w1004 -> [_ _]
          tunnel: w1003 -> [_ _]
          tunnel: w1002 -> [_ _]
          tunnel: w1001 -> [_ _]
          tunnel: w999 -> [w1022 w1041]
          tunnel: [w1027 w1039] -> w998
          tunnel: [w1024 w1036] -> w996
          tunnel: [w1023 w1037] -> w995
          tunnel: w984 -> [_ w1034]
          tunnel: w982 -> [_ w1033]
          tunnel: w981 -> [_ w1032]
          frame False {
            n523 = call "set_status_string.vi"("error in"=w1025, "new line?"=TRUE, "status string in"="Break-in Failed!", "controls array"=w1022) -> ("error out"=w1024:errorcluster, "controls array out"=w1023:refnum<vi>[])  [unwired: 6 in]
          }
          frame True {
            # "blow out cell?"
            n524 = call "run_repeatingMembraneTest_pharmabot.vi"("ExpPhase"="preQC", "error in"=w1044, "data in"=w1047, "misc common.stop memtest"=w1034, "controls array in"=w1041) -> ("error out"=w1031:errorcluster, "data out"=w1045:T9, "control array out"=w1046:refnum<vi>[])  [unwired: 2 in, 2 out]
            n525 = call "mclamp_zero_pipetteCap.vi"("error in (no error)"=w1031, "Error in"=w1032, "Multiclamp Handle Out"=w1033) -> ("error out"=w1030:errorcluster, "slow comp (pF)"=w1028:dbl, "fast comp (pF)"=w1029:dbl)  [unwired: 6 in]
            n526 = local write "slow comp (pF)"(w1028) -> ()
            n527 = local write "fast comp (pF)"(w1029) -> ()
            n528 = call "run_repeatingMembraneTest_pharmabot.vi"("ExpPhase"="preExp", "error in"=w1030, "data in"=w1045, "misc common.stop memtest"=w1034, "controls array in"=w1046) -> ("error out"=w1042:errorcluster, "data out"=w1040:T9, "control array out"=w1043:refnum<vi>[])  [unwired: 2 in, 2 out]
            n529 = call "Time Delay2"("error in (no error)"=w1042, "Delay Time (s)"=120.0) -> ("error out"=w1038:errorcluster)  [unwired: 9 in]
            n530 = call "run_repeatingMembraneTest_pharmabot.vi"("ExpPhase"="postExp", "error in"=w1038, "data in"=w1040, "misc common.stop memtest"=w1034, "controls array in"=w1043) -> ("error out"=w1036:errorcluster, "data out"=w1039:T9, "control array out"=w1037:refnum<vi>[])  [unwired: 2 in, 2 out]
          }
        }
        n531 = call "set_status_string.vi"("error in"=w996, "new line?"=TRUE, "status string in"="~~~AUTO RUN DONE~~~", "controls array"=w995) -> ("error out"=w1014:errorcluster, "controls array out"=w1015:refnum<vi>[])  [unwired: 6 in]
        n532 = Unbundle By Name(w998) -> ("experiment day folder"=w988:path, "trial name"=w987:string)
        n533 = Build Path(base path=w988, name or relative path=w987) -> (appended path=w983:path)
        n534 = call "condition_control_array.vi"("error in"=w1014, "control array in"=w1015) -> ("error out"=w985:errorcluster, "control array out"=w986:refnum<vi>[])  [unwired: 8 in]
        n535 = Build Path(base path=w983, name or relative path="config.ini") -> (appended path=w989:path)
        n536 = call "Read and Write Controls to Automatic Config File.vi"("Action"=RWC_Actions."Write", "error in"=w985, "Control References"=w986, "filepath"=w989) -> ("error out"=w994:errorcluster)  [unwired: 7 in]
        n537 = flat-sequence {
          tunnel: w994 -> [w1065]
          tunnel: [w1065] -> w993
          tunnel: [w1064] -> w992
          tunnel: w983 -> [w1053]
          frame #0 {
            w1063 = FALSE ("Experiment Done")
            w1064 = TRUE ("Experiment Done")
            n538 = Build Path(base path=w1053, name or relative path="status.txt") -> (appended path=w1061:path)
            n539 = control-ref of="status"() -> (w1052:refnum<vi>)
            n540 = local write "auto WC run trigger"(w1063) -> ()
            n541 = local write "Experiment Done"(w1064) -> ()
            n542 = local write "Running"(w1063) -> ()
            n543 = property class="Str"(reference=w1052) -> ("Value"=w1051:string)  [unwired: 1 in, 2 out]
            n544 = Open/Create/Replace File(file path (use dialog)=w1061, operation (0:open)=T33."replace or create", access (0:read/write)=enum16{"read/write", "read-only", "write-only"}."read/write") -> (refnum out=w1057:refnum<file>, error out=w1058:errorcluster)  [unwired: 3 in, 1 out]
            n545 = Write to Text File(file (use dialog)=w1057, text=w1051, error in=w1058) -> (refnum out=w1055:refnum<file>, error out=w1056:errorcluster)  [unwired: 1 in, 1 out]
            n546 = Wait (ms)(milliseconds to wait=u32 1000) -> ()  [unwired: 1 out]
            n547 = Close File(refnum=w1055, error in=w1056) -> ()  [unwired: 2 out]
          }
        }
      }
    }
    n548 = Or(x=w964, y="stop") -> (x .or. y?=w966:bool)
    n549 = Wait (ms)(milliseconds to wait=u32 50) -> ()  [unwired: 1 out]
  }
  "error out" <- w44
  "config file" <- "protocol config"
